vi "PUDELstat App.vi"() -> ()   [LabVIEW 2022 SP3]
doc: "PUDELstat App: a LabVIEW-based application to interface with and run electrochemistry experiments on the Potentiostat for Undergraduate-Designed Electrochemistry Laboratories. For more information, please visit www.eNanoLab.com/PUDELstat"
uses:
  Start.xctl
  Method Descriptions.xctl
  <vilib>/MakerHub/LINX/Public/Peripherals/PWM/PWM Set Duty Cycle 1 Chan.vi
  <vilib>/MakerHub/LINX/Public/Peripherals/Digital/Digital Read 1 Chan.vi
  <vilib>/MakerHub/LINX/Public/Peripherals/Digital/Digital Read N Chans.vi
  <vilib>/MakerHub/LINX/Private/Local IO/LinxDigitalRead.vi
  <vilib>/MakerHub/LINX/Public/Utilities/Check Channel.vi
  <vilib>/MakerHub/LINX/Public/Utilities/Open Serial.vi
  <vilib>/MakerHub/LINX/Public/Peripherals/PWM/PWM Set Duty Cycle N Chans.vi
  <vilib>/MakerHub/LINX/Private/Utilties/Generate Error.vi
  <vilib>/Utility/file.llb/Read Delimited Spreadsheet (DBL).vi
  <vilib>/Utility/file.llb/Write Delimited Spreadsheet (string).vi
  <vilib>/Utility/file.llb/Write Delimited Spreadsheet (DBL).vi
  <vilib>/MakerHub/LINX/LMH-LINX.lvlib
  <vilib>/Analysis/NI_AALPro.lvlib
panel:
  in  "Method Descriptions":bool(xcontrol)
  out "time (min)":dbl format="%#.1f"
  out "max time (min)":dbl format="%#.1f"
  out "Progress":dbl(slide) scale=0.0..30.1
  out "Current Limit":cluster{dbl, dbl}(slide)={0.001, 0.0} scale=-5.0..5.0 scale format="%_1f"
  in  "Save Path":path=path "C:/PUDELstat Data"
  in  "Method Selector":T1(tab)
  in  "Duration (s)\n[OCP]":dbl=30.0
  out "Open Circuit":cluster{dbl[], dbl[]}(graph)
  out "OCP (V)":dbl format="%#.2f"
  in  "Resolution (ms)\n[OCP]":dbl=100.0
  in  "Resolution (V)\n[CV]":dbl=0.02
  out "i (mA)\n[CV]":dbl format="%.2g"
  in  "Scan Rate (V/s)\n[CV]":dbl=0.1
  in  "Initial Potential (V)\n[CV]":dbl
  in  "First Vertex Potential (V)\n[CV]":dbl=1.0
  in  "Second Vertex Potential (V)\n[CV]":dbl=-1.0
  in  "Cycles\n[CV]":i32=1
  out "E (V)\n[CV]":dbl format="%.2g"
  out "Cyclic Voltammagram":cluster{dbl[], dbl[]}(graph)
  out "Applied and Response (CV)":T2(graph)
  in  "Final  Potential (V)\n[LSV]":dbl=1.0
  in  "Initial Potential (V)\n[LSV]":dbl
  in  "Scan Rate (V/s)\n[LSV]":dbl=0.1
  out "E (V)\n[lsv]":dbl format="%.2f"
  out "i (mA)\n[LSV]":dbl format="%.2f"
  out "Linear Sweep Voltammagram":cluster{dbl[], dbl[]}(graph)
  in  "Resolution (V)\n[LSV]":dbl=0.02
  out "Applied and Response (LSV)":T2(graph)
  in  "Scan Rate (V/s)\n[ASV]":dbl=0.1
  in  "Time (s)\n(standby)":dbl=30.0
  in  "Potential (V)\n(standby)":dbl
  in  "Final (V)\n[ASV]":dbl
  in  "Resolution (V)\n[ASV]":dbl=0.02
  in  "Time (s)\n(dep)":dbl=60.0
  in  "Potential (V)\n(dep)":dbl=-1.0
  in  "Time (s)\n(cleaning)":dbl=30.0
  in  "Potential (V)\n(cleaning)":dbl
  in  "Initial (V)\n[ASV)":dbl=-1.0
  out "Applied and Response (ASV)":T2(graph)
  out "E (V)\n[ASV]":dbl format="%.2f"
  out "i (mA)\n[ASV]":dbl format="%.2f"
  out "Anodic Stripping\n Voltammagram":cluster{dbl[], dbl[]}(graph)
  in  "Resolution (ms)\n[CA]":dbl=200.0
  out "i (mA)\n[CA]":dbl format="%.2f"
  out "q (C)":dbl format="%.2f"
  in  "Duration (s)\n[CA]":dbl=30.0
  in  "Set Potential (V)\n[CA]":dbl format="%#_13g"
  out "Chronoamperometry":cluster{dbl[], dbl[]}(graph)
  out "Energy Delivered (J)\n[CP]":dbl format="%.2f"
  out "P (mW)\n[CP]":dbl format="%.2f"
  in  "Potential (V)\n[CP]":dbl
  in  "Resolution (ms)\n[CP]":dbl=200.0
  out "E (V)\n[CP]":dbl format="%.2f"
  out "q (C)\n[CP]":dbl format="%.2f"
  in  "Duration (s)\n[CP]":dbl=10000.0
  in  "Set Current (mA)\n[CP]":dbl format="%#_13g"
  out "Chronopotentiometry":cluster{dbl[], dbl[]}(graph)
  out "E (V)\n[GC]":dbl format="%.2f"
  out "Galvanostatic Cycling":cluster{dbl[], dbl[]}(graph)
  in  "Set Current (mA)\n[GC]":dbl=5.0 format="%#_13g"
  in  "Duration (s)\n[GC]":dbl=30.0
  in  "Resolution (ms)\n[CP] 2":dbl=100.0
  in  "Measure Ru":bool=TRUE
  out "Ru (Ohm)":dbl format="%#.1f"
  in  "% Compensation":dbl=85.0
  out "Rc (Ohm)":dbl format="%#.1f"
  out "Eap (V)\n[iR]":dbl format="%.2f"
  out "i (mA)\n[iR]":dbl format="%.2f"
  in  "Cycles\n[iR]":i32=100
  in  "Pertubation Potential (V)":dbl=0.25
  in  "Resting Potential (V)":dbl format="%#_13g"
  in  "Frequency (mHz)\n[iR]":dbl=500.0 format="%#_13g"
  in  "Resolution (ms)\n[iR]":dbl=50.0
  out "Applied and Response (Ohmic)":T2(graph)
  in  "Potential Calibration":dbl[][](array[numeric])=[[0.954619, 0.02673]]
  in  "Current Calibration":dbl[][](array[numeric])=[[220.0, 4.99643, 0.11518, -10.0, 10.0], [510.0, 2.18568, 0.06108, -5.0, 5.0], [1000.0, 1.18065, 0.04067, -2.75, 2.75], [10000.0, 0.203334, 0.0077, -0.5, 0.5]]
  out "E Offset\n[Cal]":dbl format="%0.5f"
  out "R²\n[Calib] E":dbl format="%#_6f"
  out "E Conversion":dbl format="%#_6f"
  out "E Calibration":T3(graph)
  out "i Offset\n[Cal]":dbl format="%0.5f"
  out "R²\n[Calib] i":dbl format="%#_6f"
  out "i Conversion":dbl format="%#_6f"
  out "i Calibration":T3(graph)
  in  "Cycles \n[Cal]":i32=1
  in  "E2 (V)\n[Cal]":dbl=-1.0
  in  "E1 (V)\n[Cal]":dbl=1.0
  in  "Ei (V)\n[Cal]":dbl
  in  "Scan Rate (V/s)\n[Cal]":dbl=0.1
  in  "Sample Cell  Resistance (Ohm)":dbl=1000.0
  in  "Resolution (ms)\n[Cal]":dbl=100.0
  out "Applied and Response (Cal)":T2(graph)
  in  "Save Plot":u16(ring) items=["i vs E", "i vs t"]
  out "Preview (Single Cycle)":cluster{dbl[], "Preview":dbl[]}[](graph)
  in  "Element Selector":enum32{"A", "B", "C", "D", "E"}(tab) caption="Elements"
  in  "Input A":T4={"Element A"=0, "Scan Rate A"={"DE (V)\n[A]"=0.2, "Dt (s)\n[A]"=1.0}, "Input--Timing A"={"Duration (s)\n[MB-A]"=30.0, "Sample Rate (ms)\n[MB-A]"=100.0, "Frequency (mHz)\n[MB-A]"=1000.0, "Repeat n Times\n[MB-A]"=0}, "Input--Potential A"={"Ei (V)\n[A]"=0.0, "Ef (V)\n[A]"=1.0, "E1 (V)\n[A]"=1.0, "E2 (V)\n[A]"=-1.0, "Duty Cycle (%)\n[A]"=50.0}} {"Scan Rate A"."Dt (s)\n[A]" format="%0.2f"; "Scan Rate A"."DE (V)\n[A]" format="%0.2f"; "Element A" items=["Disabled", "Potentiostatic", "Linear Ramp", "Staircase Ramp", "Triangle Wave", "Square Wave", "Staircase Wave", "Sine Wave"]}
  in  "Input B":T5={"Element B"=0, "Input--Potential B"={"Ei (V)\n[B]"=0.0, "Ef (V)\n[B]"=1.0, "E1 (V)\n[B]"=1.0, "E2 (V)\n[B]"=-1.0, "Duty Cycle (%)\n[B]"=50.0}, "Input--Timing B"={"Duration (s)\n[MB-B]"=30.0, "Sample Rate (ms)\n[MB-B]"=100.0, "Frequency (mHz)\n[MB-B]"=1000.0, "Repeat n Times\n[MB-B]"=0}, "Scan Rate B"={"DE (V)\n[B]"=0.2, "Dt (s)\n[B]"=1.0}} {"Scan Rate B"."Dt (s)\n[B]" format="%0.2f"; "Scan Rate B"."DE (V)\n[B]" format="%0.2f"; "Element B" items=["Disabled", "Potentiostatic", "Linear Ramp", "Staircase Ramp", "Triangle Wave", "Square Wave", "Staircase Wave", "Sine Wave"]}
  in  "Input C":T6={"Scan Rate C"={"DE (V)\n[C]"=0.2, "Dt (s)\n[C]"=1.0}, "Input--Timing C"={"Duration (s)\n[MB-C]"=30.0, "Sample Rate (ms)\n[MB-C]"=100.0, "Frequency (mHz)\n[MB-C]"=1000.0, "Repeat n Times\n[MB-C]"=0}, "Input--Potential C"={"Ei (V)\n[C]"=0.0, "Ef (V)\n[C]"=1.0, "E1 (V)\n[C]"=1.0, "E2 (V)\n[C]"=-1.0, "Duty Cycle (%)\n[C]"=50.0}, "Element C"=0} {"Scan Rate C"."Dt (s)\n[C]" format="%0.2f"; "Scan Rate C"."DE (V)\n[C]" format="%0.2f"; "Element C" items=["Disabled", "Potentiostatic", "Linear Ramp", "Staircase Ramp", "Triangle Wave", "Square Wave", "Staircase Wave", "Sine Wave"]}
  in  "Input D":T7={"Scan Rate D"={"DE (V)\n[D]"=0.2, "Dt (s)\n[D]"=1.0}, "Input--Timing D"={"Duration (s)\n[MB-D]"=30.0, "Sample Rate (ms)\n[MB-D]"=100.0, "Frequency (mHz)\n[MB-D]"=1000.0, "Repeat n Times\n[MB-D]"=0}, "Input--Potential D"={"Ei (V)\n[D]"=0.0, "Ef (V)\n[D]"=1.0, "E1 (V)\n[D]"=1.0, "E2 (V)\n[D]"=-1.0, "Duty Cycle (%)\n[D]"=50.0}, "Element D"=0} {"Scan Rate D"."Dt (s)\n[D]" format="%0.2f"; "Scan Rate D"."DE (V)\n[D]" format="%0.2f"; "Element D" items=["Disabled", "Potentiostatic", "Linear Ramp", "Staircase Ramp", "Triangle Wave", "Square Wave", "Staircase Wave", "Sine Wave"]}
  in  "Input E":T8={"Scan Rate E"={"DE (V)\n[E]"=0.2, "Dt (s)\n[E]"=1.0}, "Input--Timing E"={"Duration (s)\n[MB-E]"=30.0, "Sample Rate (ms)\n[MB-E]"=100.0, "Frequency (mHz)\n[MB-E]"=1000.0, "Repeat n Times\n[MB-E]"=0}, "Input--Potential E"={"Ei (V)\n[E]"=0.0, "Ef (V)\n[E]"=1.0, "E1 (V)\n[E]"=1.0, "E2 (V)\n[E]"=-1.0, "Duty Cycle (%)\n[E]"=50.0}, "Element E"=0} {"Scan Rate E"."Dt (s)\n[E]" format="%0.2f"; "Scan Rate E"."DE (V)\n[E]" format="%0.2f"; "Element E" items=["Disabled", "Potentiostatic", "Linear Ramp", "Staircase Ramp", "Triangle Wave", "Square Wave", "Staircase Wave", "Sine Wave"]}
  in  "Mode":u16(ring) items=["Sequence: A->B->C->D->E", "Superimpose: A + B"]
  in  "Cycles\n[MB]":i32=1
  out "Signal Frequencies (mHz)":cluster{"A":dbl, "B":dbl}
  out "E (V)\nMB":dbl format="%.2f"
  out "i (mA)\n[MB]":dbl format="%.2f"
  out "Method i-t":cluster{dbl[], dbl[]}(graph)
  out "Method i-E":cluster{dbl[], dbl[]}(graph)
  out "R² \n[analysis]":dbl format="%#_6f"
  in  "Open Data":path
  in  "Plot Type":u16(ring) items=["Linear", "Tafel"]
  in  "E0 (V vs ref)":dbl
  out "Tafel Slope (mV/decade)":dbl
  out "i0 (mA)":dbl
  out "Analysis":cluster{"all rows":dbl[], "all rows":dbl[]}[](graph)
  in  "Cycle":dbl(ring)
  in  "Sensitivity (Jumper)":u16(ring)=1 items=["± 10 mA (220 Ohm)", "± 5 mA (510 Ohm)", "± 2.75 mA (1 kOhm)", "± 0.5 mA (10 kOhm)"]
  in  "Serial Port":refnum<visa-resource-name>="COM3"
  in  "Start":bool(xcontrol)
  in  "stop":bool
  # "/"
  # "(min)"
  # "Current Limits"
  # "Cleaning Step:"
  # "Deposition Step:"
  # "Stripping Step:"
  # "Standby:"
  # "Stop Condition:"
  # "or"
  # "E Conversion (measured/control)"
  # "E Offset (V)"
  # "Jumper (W)"
  # "i Conversion (mA/V)"
  # "i Offset (mA)"
  # "mHz"
  # "mHz"
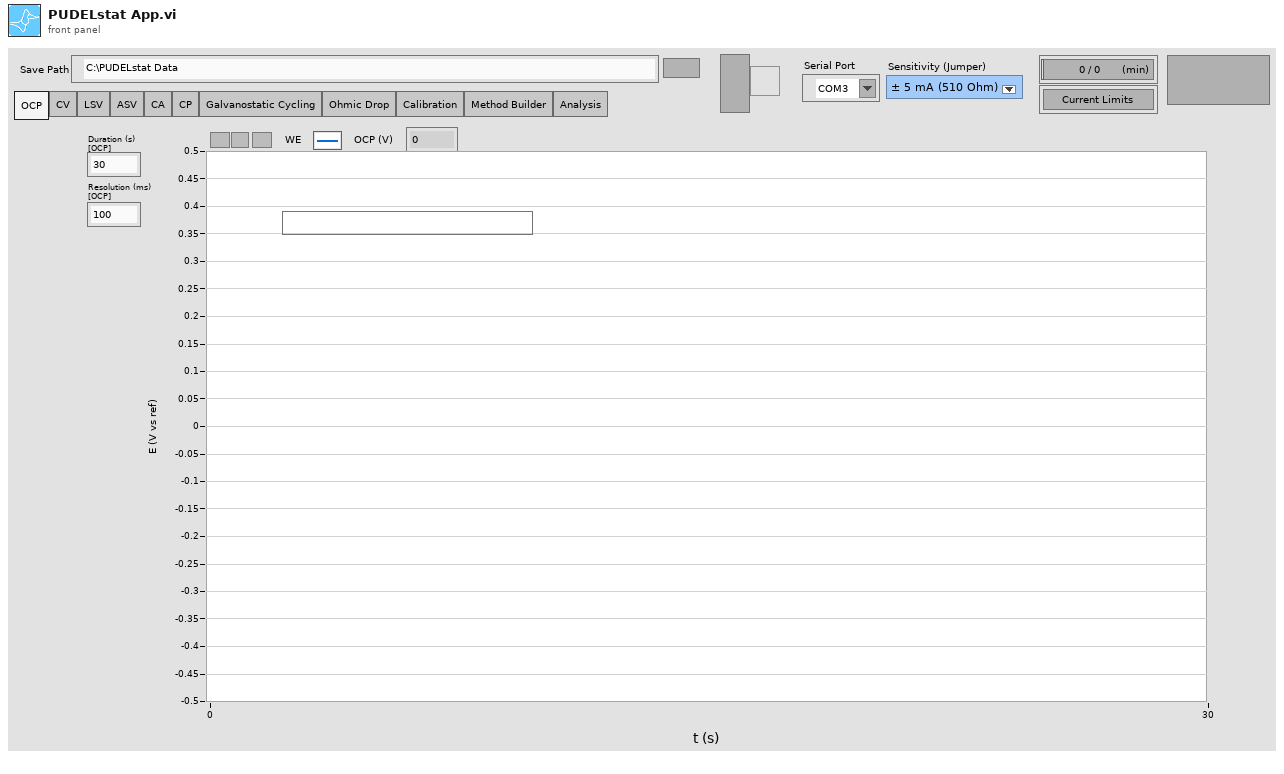
[diagram p1: front panel]
types:
  T1 = enum32{"OCP", "CV", "LSV", "ASV", "CA", "CP", "Galvanostatic Cycling", "Ohmic Drop", "Calibration", "Method Builder", "Analysis"}
  T2 = cluster{"Elapsed Time (s)":dbl[], "i (mA)":dbl[]}[]
  T3 = cluster{"Elapsed Time (s)":dbl[], "Best Linear Fit":dbl[]}[]
  T4 = cluster{"Element A":u16, "Scan Rate A":cluster{"DE (V)\n[A]":dbl, "Dt (s)\n[A]":dbl}, "Input--Timing A":cluster{"Duration (s)\n[MB-A]":dbl, "Sample Rate (ms)\n[MB-A]":dbl, "Frequency (mHz)\n[MB-A]":dbl, "Repeat n Times\n[MB-A]":i32}, "Input--Potential A":cluster{"Ei (V)\n[A]":dbl, "Ef (V)\n[A]":dbl, "E1 (V)\n[A]":dbl, "E2 (V)\n[A]":dbl, "Duty Cycle (%)\n[A]":dbl}}
  T5 = cluster{"Element B":u16, "Input--Potential B":cluster{"Ei (V)\n[B]":dbl, "Ef (V)\n[B]":dbl, "E1 (V)\n[B]":dbl, "E2 (V)\n[B]":dbl, "Duty Cycle (%)\n[B]":dbl}, "Input--Timing B":cluster{"Duration (s)\n[MB-B]":dbl, "Sample Rate (ms)\n[MB-B]":dbl, "Frequency (mHz)\n[MB-B]":dbl, "Repeat n Times\n[MB-B]":i32}, "Scan Rate B":cluster{"DE (V)\n[B]":dbl, "Dt (s)\n[B]":dbl}}
  T6 = cluster{"Scan Rate C":cluster{"DE (V)\n[C]":dbl, "Dt (s)\n[C]":dbl}, "Input--Timing C":cluster{"Duration (s)\n[MB-C]":dbl, "Sample Rate (ms)\n[MB-C]":dbl, "Frequency (mHz)\n[MB-C]":dbl, "Repeat n Times\n[MB-C]":i32}, "Input--Potential C":cluster{"Ei (V)\n[C]":dbl, "Ef (V)\n[C]":dbl, "E1 (V)\n[C]":dbl, "E2 (V)\n[C]":dbl, "Duty Cycle (%)\n[C]":dbl}, "Element C":u16}
  T7 = cluster{"Scan Rate D":cluster{"DE (V)\n[D]":dbl, "Dt (s)\n[D]":dbl}, "Input--Timing D":cluster{"Duration (s)\n[MB-D]":dbl, "Sample Rate (ms)\n[MB-D]":dbl, "Frequency (mHz)\n[MB-D]":dbl, "Repeat n Times\n[MB-D]":i32}, "Input--Potential D":cluster{"Ei (V)\n[D]":dbl, "Ef (V)\n[D]":dbl, "E1 (V)\n[D]":dbl, "E2 (V)\n[D]":dbl, "Duty Cycle (%)\n[D]":dbl}, "Element D":u16}
  T8 = cluster{"Scan Rate E":cluster{"DE (V)\n[E]":dbl, "Dt (s)\n[E]":dbl}, "Input--Timing E":cluster{"Duration (s)\n[MB-E]":dbl, "Sample Rate (ms)\n[MB-E]":dbl, "Frequency (mHz)\n[MB-E]":dbl, "Repeat n Times\n[MB-E]":i32}, "Input--Potential E":cluster{"Ei (V)\n[E]":dbl, "Ef (V)\n[E]":dbl, "E1 (V)\n[E]":dbl, "E2 (V)\n[E]":dbl, "Duty Cycle (%)\n[E]":dbl}, "Element E":u16}
  T9 = typedef "LMH-LINX.lvlib/LINX Ref.ctl" = cluster{"IO":T10, "Interface":T11, "LINX Device Config":T12}
  T10 = typedef "LMH-LINX.lvlib/Platform.ctl" = enum16{"Remote", "Local"}
  T11 = typedef "LMH-LINX.lvlib/Interface.ctl" = enum16{"Serial", "TCP"}
  T12 = typedef "LMH-LINX.lvlib/Device.lvlib/LINX Device Config.ctl" = cluster{"Interface":T11, "COM Port":refnum<visa-resource-name>, "TCP Configuration":T13, "Device Family":u8, "Device ID":u8, "Device Name":string, "TCP Ref":refnum<k5>, "Channels":T14}
  T13 = typedef "LMH-LINX.lvlib/Device.lvlib/TCP Config.ctl" = cluster{"IP Address":string, "Port":u16}
  T14 = typedef "LMH-LINX.lvlib/Channels.ctl" = cluster{"DI":u8[], "DO":u8[], "AI":u8[], "AO":u8[], "PWM":u8[], "QE":u8[], "UART":u8[], "I2C 2":u8[], "SPI":u8[], "CAN":u8[], "Servo":u8[], "AI Ref (V)":dbl, "AI Resolution (Bits)":u8, "AO Ref (V)":dbl, "AO Resolution (Bits)":u8}
  T15 = cluster{"Error Out":errorcluster, "LINX Resource":T9}
  T16 = cluster{"Signal Averaging?":bool, "CA?":bool, "Step Width":dbl}
  T17 = enum16{"Disabled", "Potentiostatic", "Linear Ramp", "Staircase Ramp", "Triangle Wave", "Square Wave", "Staircase Wave", "Sine Wave"}
  T18 = cluster{"Scan Rate D":cluster{"DE (V)":dbl, "Dt (s)":dbl}, "Input--Timing D":cluster{"Duration (s)":dbl, "Sample Rate (ms)":dbl, "Frequency (mHz)":dbl, "Repeat n Times":i32}, "Input--Potential D":cluster{"Ei (V)":dbl, "Ef (V)":dbl, "E1 (V)":dbl, "E2 (V)":dbl, "Duty Cycle (%)":dbl}, "Element D":u16}
  T19 = cluster{"Scan Rate C":cluster{"DE (V)":dbl, "Dt (s)":dbl}, "Input--Timing C":cluster{"Duration (s)":dbl, "Sample Rate (ms)":dbl, "Frequency (mHz)":dbl, "Repeat n Times":i32}, "Input--Potential C":cluster{"Ei (V)":dbl, "Ef (V)":dbl, "E1 (V)":dbl, "E2 (V)":dbl, "Duty Cycle (%)":dbl}, "Element C":u16}
  T20 = cluster{"Element B":u16, "Input--Potential B":cluster{"Ei (V)":dbl, "Ef (V)":dbl, "E1 (V)":dbl, "E2 (V)":dbl, "Duty Cycle (%)":dbl}, "Input--Timing B":cluster{"Duration (s)":dbl, "Sample Rate (ms)":dbl, "Frequency (mHz)":dbl, "Repeat n Times":i32}, "Scan Rate B":cluster{"DE (V)":dbl, "Dt (s)":dbl}}
  T21 = cluster{"Element A":u16, "Scan Rate A":cluster{"DE (V)":dbl, "Dt (s)":dbl}, "Input--Timing A":cluster{"Duration (s)":dbl, "Sample Rate (ms)":dbl, "Frequency (mHz)":dbl, "Repeat n Times":i32}, "Input--Potential A":cluster{"Ei (V)":dbl, "Ef (V)":dbl, "E1 (V)":dbl, "E2 (V)":dbl, "Duty Cycle (%)":dbl}}
  T22 = cluster{"Duty Cycle Array":dbl[], "Wait Time (ms)":dbl, "Array Size":i32, "Frequency (mHz)":dbl, "Corrected Duty Cycle Array":dbl[], "Potential Array":dbl[]}
  T23 = cluster{dbl[], "Resolution (ms)\n[OCP]":dbl, i32, dbl, dbl[], dbl[]}
  T24 = cluster{"Initial Potential (V)\n[CV]":dbl, dbl, "First Vertex Potential (V)\n[CV]":dbl, "Second Vertex Potential (V)\n[CV]":dbl, dbl}
  T25 = cluster{"Initial Potential (V)\n[LSV]":dbl, "Final  Potential (V)\n[LSV]":dbl, dbl, dbl, dbl}
  T26 = cluster{"Duration (s)\n[CA]":dbl, "Resolution (ms)\n[CA]":dbl, dbl, i32}
  T27 = cluster{"Set Potential (V)\n[CA]":dbl, dbl, dbl, dbl, dbl}
  T28 = cluster{"Duration (s)\n[CP]":dbl, "Resolution (ms)\n[CP]":dbl, dbl, i32}
  T29 = cluster{"Resting Potential (V)":dbl, "Pertubation Potential (V)":dbl, dbl, dbl, dbl}
  T30 = cluster{dbl, "Resolution (ms)\n[iR]":dbl, "Frequency (mHz)\n[iR]":dbl, i32}
  T31 = cluster{"Ei (V)\n[Cal]":dbl, dbl, "E1 (V)\n[Cal]":dbl, "E2 (V)\n[Cal]":dbl, dbl}
  T32 = cluster{dbl, "Resolution (ms)\n[Cal]":dbl, dbl, i32}
  T33 = cluster{"Elapsed Time (s)":dbl[], "E (V)":dbl[], "i (mA)":dbl[], "Vr (V)":dbl[], "Eraw (V)":dbl[]}
  T34 = cluster{"Wait Time (ms)":dbl, i32, "Array Size":i32, u32}
  T35 = cluster{"Elapsed Time (s)":dbl[], "i (mA)":dbl[]}
  T36 = cluster{"Elapsed Time (s)":dbl[], "Eraw (V)":dbl[]}
  T37 = cluster{"error out":errorcluster, "LINX Resource out":T9}
  T38 = cluster{"E (V)":dbl[], "Best Linear Fit":dbl[]}[]
  T39 = cluster{"Eraw (V)":dbl[], "Best Linear Fit":dbl[]}
  T40 = cluster{"Eraw (V)":dbl[], "Best Linear Fit":dbl[]}[]
  T41 = cluster{"error out":errorcluster, "LINX Resource":T9}
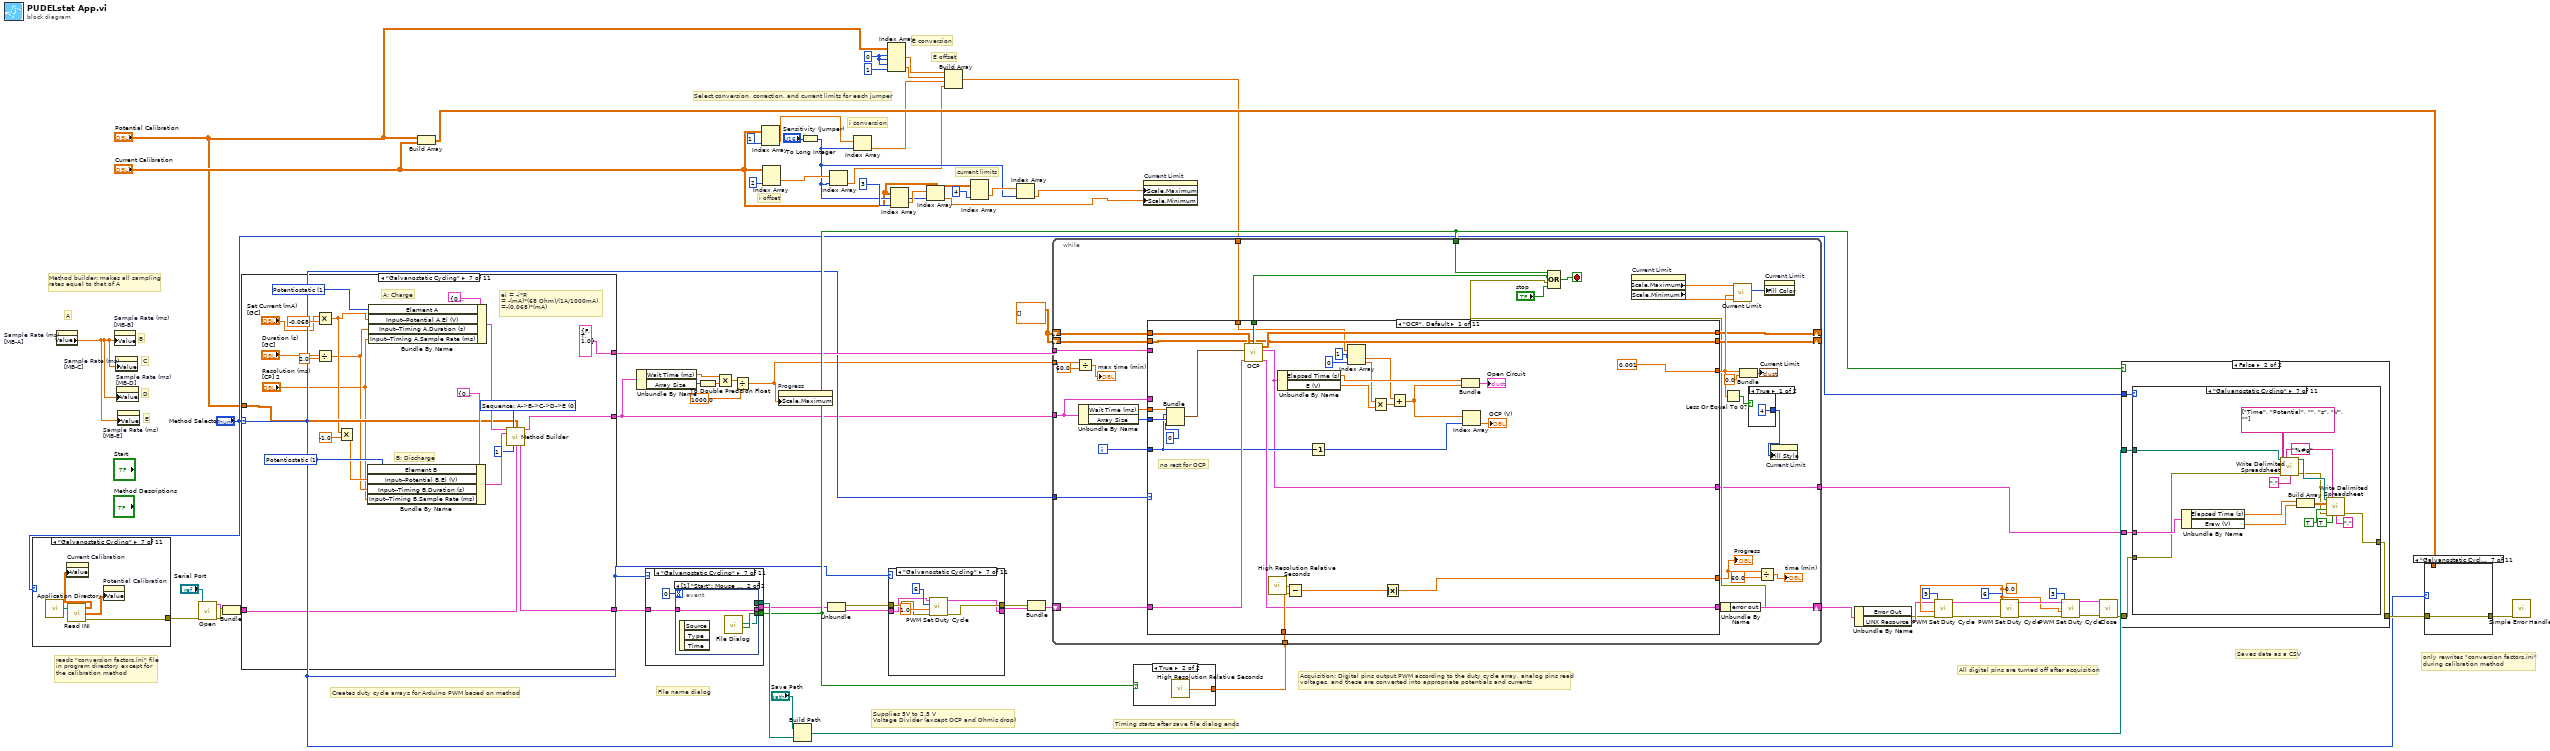
[diagram p0: block diagram]
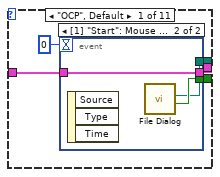
[diagram p2: hidden frame]
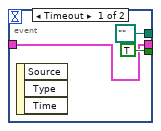
[diagram p3: hidden frame]
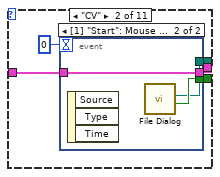
[diagram p4: hidden frame]
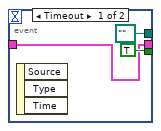
[diagram p5: hidden frame]
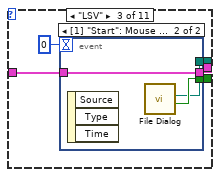
[diagram p6: hidden frame]
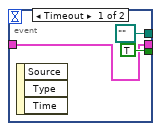
[diagram p7: hidden frame]
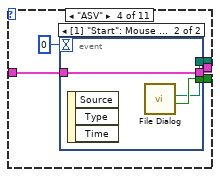
[diagram p8: hidden frame]
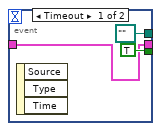
[diagram p9: hidden frame]
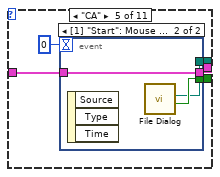
[diagram p10: hidden frame]
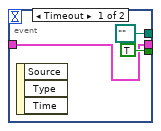
[diagram p11: hidden frame]
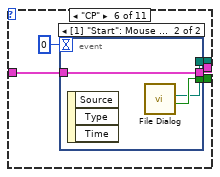
[diagram p12: hidden frame]
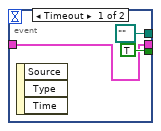
[diagram p13: hidden frame]
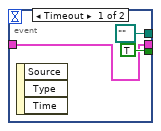
[diagram p14: hidden frame]
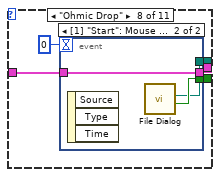
[diagram p15: hidden frame]
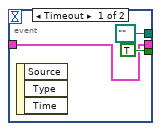
[diagram p16: hidden frame]
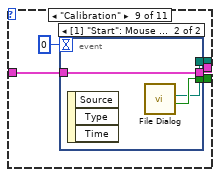
[diagram p17: hidden frame]
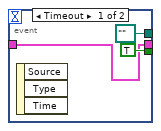
[diagram p18: hidden frame]
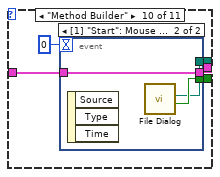
[diagram p19: hidden frame]
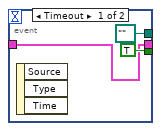
[diagram p20: hidden frame]
diagram:
  w7 = 0 ("index (row)")
  w29 = dbl[][] [] ("Data Out")
  w46 = 0.0 ("Duty Cycle (0-1)")
  # "E offset"
  # "E conversion"
  # "current limits"
  # "i offset"
  # "i conversion"
  # "Select conversion, correction, and current limits for each jumper"
  # "Saves data as a CSV"
  # "All digital pins are turned off after acquisition"
  # "Acquisition: Digital pins output PWM according to the duty cycle array, analog pins read\nvoltages, and these are converted into appropriate potentials and currents"
  # "File name dialog"
  # "Creates duty cycle arrays for Arduino PWM based on method"
  # "Supplies 5V to 2.5 V\nVoltage Divider (except OCP and Ohmic drop)"
  # "only rewrites \"conversion factors.ini\"\nduring calibration method"
  # "reads \"conversion factors.ini\" file\nin program directory except for\nthe calibration method"
  # "Timing starts after save file dialog ends"
  # "Method builder: makes all sampling\nrates equal to that of A"
  # "E"
  # "D"
  # "C"
  # "B"
  # "A"
  n1 = case shown="\"Galvanostatic Cycling\"" "Method Selector" {
    tunnel: [w69 w73 w77 w81 w85 w89 w93 w97 errorcluster {"status"=FALSE, "code"=0, "source"=""} ("error out") w102 w106] -> w32
    frame "OCP", Default {
      n2 = call <vilib>:"Application Directory.vi"() -> ("Application Directory"=w70:path)
      n3 = call "Read INI.vi"("Path"=w70) -> ("Current Calibration"=w71:dbl[][], "Voltage Calibration"=w68:dbl[][], "error out"=w69:errorcluster)  [unwired: 1 in]
      n4 = property on="Current Calibration" class="Arr (strict)"("Value"=w71) -> ()  [unwired: 2 in, 2 out]
      n5 = property on="Potential Calibration" class="Arr (strict)"("Value"=w68) -> ()  [unwired: 2 in, 2 out]
    }
    frame "CV" {
      n6 = call <vilib>:"Application Directory.vi"() -> ("Application Directory"=w74:path)
      n7 = call "Read INI.vi"("Path"=w74) -> ("Current Calibration"=w75:dbl[][], "Voltage Calibration"=w72:dbl[][], "error out"=w73:errorcluster)  [unwired: 1 in]
      n8 = property on="Current Calibration" class="Arr (strict)"("Value"=w75) -> ()  [unwired: 2 in, 2 out]
      n9 = property on="Potential Calibration" class="Arr (strict)"("Value"=w72) -> ()  [unwired: 2 in, 2 out]
    }
    frame "LSV" {
      n10 = call <vilib>:"Application Directory.vi"() -> ("Application Directory"=w78:path)
      n11 = call "Read INI.vi"("Path"=w78) -> ("Current Calibration"=w79:dbl[][], "Voltage Calibration"=w76:dbl[][], "error out"=w77:errorcluster)  [unwired: 1 in]
      n12 = property on="Current Calibration" class="Arr (strict)"("Value"=w79) -> ()  [unwired: 2 in, 2 out]
      n13 = property on="Potential Calibration" class="Arr (strict)"("Value"=w76) -> ()  [unwired: 2 in, 2 out]
    }
    frame "ASV" {
      n14 = call <vilib>:"Application Directory.vi"() -> ("Application Directory"=w82:path)
      n15 = call "Read INI.vi"("Path"=w82) -> ("Current Calibration"=w83:dbl[][], "Voltage Calibration"=w80:dbl[][], "error out"=w81:errorcluster)  [unwired: 1 in]
      n16 = property on="Current Calibration" class="Arr (strict)"("Value"=w83) -> ()  [unwired: 2 in, 2 out]
      n17 = property on="Potential Calibration" class="Arr (strict)"("Value"=w80) -> ()  [unwired: 2 in, 2 out]
    }
    frame "CA" {
      n18 = call <vilib>:"Application Directory.vi"() -> ("Application Directory"=w86:path)
      n19 = call "Read INI.vi"("Path"=w86) -> ("Current Calibration"=w87:dbl[][], "Voltage Calibration"=w84:dbl[][], "error out"=w85:errorcluster)  [unwired: 1 in]
      n20 = property on="Current Calibration" class="Arr (strict)"("Value"=w87) -> ()  [unwired: 2 in, 2 out]
      n21 = property on="Potential Calibration" class="Arr (strict)"("Value"=w84) -> ()  [unwired: 2 in, 2 out]
    }
    frame "CP" {
      n22 = call <vilib>:"Application Directory.vi"() -> ("Application Directory"=w90:path)
      n23 = call "Read INI.vi"("Path"=w90) -> ("Current Calibration"=w91:dbl[][], "Voltage Calibration"=w88:dbl[][], "error out"=w89:errorcluster)  [unwired: 1 in]
      n24 = property on="Current Calibration" class="Arr (strict)"("Value"=w91) -> ()  [unwired: 2 in, 2 out]
      n25 = property on="Potential Calibration" class="Arr (strict)"("Value"=w88) -> ()  [unwired: 2 in, 2 out]
    }
    frame "Galvanostatic Cycling" {
      n26 = call <vilib>:"Application Directory.vi"() -> ("Application Directory"=w94:path)
      n27 = call "Read INI.vi"("Path"=w94) -> ("Current Calibration"=w95:dbl[][], "Voltage Calibration"=w92:dbl[][], "error out"=w93:errorcluster)  [unwired: 1 in]
      n28 = property on="Current Calibration" class="Arr (strict)"("Value"=w95) -> ()  [unwired: 2 in, 2 out]
      n29 = property on="Potential Calibration" class="Arr (strict)"("Value"=w92) -> ()  [unwired: 2 in, 2 out]
    }
    frame "Ohmic Drop" {
      n30 = call <vilib>:"Application Directory.vi"() -> ("Application Directory"=w98:path)
      n31 = call "Read INI.vi"("Path"=w98) -> ("Current Calibration"=w99:dbl[][], "Voltage Calibration"=w96:dbl[][], "error out"=w97:errorcluster)  [unwired: 1 in]
      n32 = property on="Current Calibration" class="Arr (strict)"("Value"=w99) -> ()  [unwired: 2 in, 2 out]
      n33 = property on="Potential Calibration" class="Arr (strict)"("Value"=w96) -> ()  [unwired: 2 in, 2 out]
    }
    frame "Calibration" {
    }
    frame "Method Builder" {
      n34 = call <vilib>:"Application Directory.vi"() -> ("Application Directory"=w103:path)
      n35 = call "Read INI.vi"("Path"=w103) -> ("Current Calibration"=w104:dbl[][], "Voltage Calibration"=w101:dbl[][], "error out"=w102:errorcluster)  [unwired: 1 in]
      n36 = property on="Current Calibration" class="Arr (strict)"("Value"=w104) -> ()  [unwired: 2 in, 2 out]
      n37 = property on="Potential Calibration" class="Arr (strict)"("Value"=w101) -> ()  [unwired: 2 in, 2 out]
    }
    frame "Analysis" {
      n38 = call <vilib>:"Application Directory.vi"() -> ("Application Directory"=w107:path)
      n39 = call "Read INI.vi"("Path"=w107) -> ("Current Calibration"=w108:dbl[][], "Voltage Calibration"=w105:dbl[][], "error out"=w106:errorcluster)  [unwired: 1 in]
      n40 = property on="Current Calibration" class="Arr (strict)"("Value"=w108) -> ()  [unwired: 2 in, 2 out]
      n41 = property on="Potential Calibration" class="Arr (strict)"("Value"=w105) -> ()  [unwired: 2 in, 2 out]
    }
  }
  n42 = property on="Sample Rate (ms)\n[MB-A]" class="DigNum (strict)"() -> ("Value"=w35:dbl)  [unwired: 2 in, 2 out]
  n43 = property on="Sample Rate (ms)\n[MB-B]" class="DigNum (strict)"("Value"=w35) -> ()  [unwired: 2 in, 2 out]
  n44 = property on="Sample Rate (ms)\n[MB-C]" class="DigNum (strict)"("Value"=w35) -> ()  [unwired: 2 in, 2 out]
  n45 = property on="Sample Rate (ms)\n[MB-D]" class="DigNum (strict)"("Value"=w35) -> ()  [unwired: 2 in, 2 out]
  n46 = property on="Sample Rate (ms)\n[MB-E]" class="DigNum (strict)"("Value"=w35) -> ()  [unwired: 2 in, 2 out]
  n47 = call-poly <vilib>:"Open.vi"("Error In"=w32, "Serial Port"="Serial Port") -> ("Error Out"=w44:errorcluster, "LINX Resource"=w43:T9)  [unwired: 7 in, 1 out]
  n48 = Bundle("Error Out"=w44, "LINX Resource"=w43) -> (w42:T15)  [unwired: 1 in]
  n49 = case shown="\"Galvanostatic Cycling\"" "Method Selector" {
    tunnel: w42 -> [w120 w140 w166 w184 w218 w232 w246 w263 w280 w296 w308]
    tunnel: [w120 w139 w165 w183 w217 w231 w247 w262 w279 w295 w308] -> w22
    tunnel: [w111 w123 w164 w173 w212 w233 w249 w264 w278 w294 T22 {"Duty Cycle Array"=[], "Wait Time (ms)"=0.0, "Array Size"=0, "Frequency (mHz)"=0.0, "Corrected Duty Cycle Array"=[], "Potential Array"=[]} ("Output")] -> w11
    tunnel: [T16 {"Signal Averaging?"=FALSE, "CA?"=FALSE, "Step Width"=1.0} ("Averaging and Conversion") w137 w162 w206 T16 {"Signal Averaging?"=FALSE, "CA?"=TRUE, "Step Width"=1.0} ("Averaging and Conversion") T16 {"Signal Averaging?"=FALSE, "CA?"=TRUE, "Step Width"=1.0} ("Averaging and Conversion") T16 {"Signal Averaging?"=FALSE, "CA?"=TRUE, "Step Width"=1.0} ("Averaging and Conversion") T16 {"Signal Averaging?"=FALSE, "CA?"=FALSE, "Step Width"=1.0} ("Averaging and Conversion") T16 {"Signal Averaging?"=FALSE, "CA?"=FALSE, "Step Width"=1.0} ("Averaging and Conversion") T16 {"Signal Averaging?"=FALSE, "CA?"=FALSE, "Step Width"=1.0} ("Averaging and Conversion") T16 {"Signal Averaging?"=FALSE, "CA?"=FALSE, "Step Width"=0.0} ("Averaging and Conversion")] -> w28
    tunnel: "Potential Calibration" -> [_ w121 w147 w174 w208 w221 w248 w258 w274 w292 _]
    frame "OCP", Default {
      w109 = dbl[] []
      # "Samples = Duration/resolution\n+1 (for spurious first pt)"
      n50 = Multiply(x=1000.0, y="Duration (s)\n[OCP]") -> (x*y=w118:dbl)
      n51 = Divide(x=w118, y="Resolution (ms)\n[OCP]") -> (x/y=w117:dbl)
      n52 = Increment(x=w117) -> (x+1=w116:dbl)
      n53 = To Long Integer(number=w116) -> (32bit integer=w113:i32)
      n54 = Bundle(w109, "Resolution (ms)\n[OCP]"="Resolution (ms)\n[OCP]", w113, 0.0, w109, w109) -> (w111:T23)  [unwired: 1 in]
    }
    frame "CV" {
      w132 = 20.0 ("Resolution (ms)")
      w124 = 0.0
      # "20 ms sampling (50 Hz)"
      n55 = Decrement(x="Cycles\n[CV]") -> (x-1=w142:i32)
      n56 = Divide(x="Resolution (V)\n[CV]", y="Scan Rate (V/s)\n[CV]") -> (x/y=w128:dbl)
      n57 = Bundle By Name(cluster=cluster{"DE (V)":dbl, "Dt (s)":dbl} {"DE (V)"=1.0, "Dt (s)"=1.0} ("Input--Scan Rate"), "DE (V)"="Resolution (V)\n[CV]", "Dt (s)"=w128) -> (w126:cluster{"DE (V)":dbl, "Dt (s)":dbl})
      n58 = Bundle("Initial Potential (V)\n[CV]"="Initial Potential (V)\n[CV]", w124, "First Vertex Potential (V)\n[CV]"="First Vertex Potential (V)\n[CV]", "Second Vertex Potential (V)\n[CV]"="Second Vertex Potential (V)\n[CV]", w124) -> (w144:T24)  [unwired: 1 in]
      n59 = Bundle(w124, "Resolution (ms)"=w132, w124, w142) -> (w141:cluster{dbl, "Resolution (ms)":dbl, dbl, i32})  [unwired: 1 in]
      n60 = Divide(x=w132, y=1000.0) -> (x/y=w133:dbl)
      n61 = Divide(x=w128, y=w133) -> (x/y=w127:dbl)
      n62 = call "Method Elements.vi"("Arduino In"=w140, "Potential Calibration"=w121, "Input--Scan Rate"=w126, "Input--Timing"=w141, "Input--Potential"=w144, "Element"=T17."Staircase Wave") -> ("Output"=w123:T22, "Arduino Out"=w139:cluster{"Error Out":errorcluster, "LINX Out":T9})  [unwired: 4 in]
      n63 = Bundle By Name(cluster=T16 {"Signal Averaging?"=TRUE, "CA?"=FALSE, "Step Width"=0.0} ("Averaging and Conversion"), "Signal Averaging?"=TRUE ("Signal Averaging? 2"), "CA?"=FALSE ("Signal Averaging? 2"), "Step Width"=w127) -> (w137:T16)
    }
    frame "LSV" {
      w151 = 20.0
      w167 = 0.0
      # "20 ms sampling (50 Hz)"
      n64 = Divide(x="Resolution (V)\n[LSV]", y="Scan Rate (V/s)\n[LSV]") -> (x/y=w152:dbl)
      n65 = Bundle(w167, w151, w167, 0) -> (w159:cluster{dbl, dbl, dbl, i32})  [unwired: 1 in]
      n66 = Bundle("Initial Potential (V)\n[LSV]"="Initial Potential (V)\n[LSV]", "Final  Potential (V)\n[LSV]"="Final  Potential (V)\n[LSV]", w167, w167, w167) -> (w169:T25)  [unwired: 1 in]
      n67 = Bundle By Name(cluster=cluster{"DE (V)":dbl, "Dt (s)":dbl} {"DE (V)"=1.0, "Dt (s)"=1.0} ("Input--Scan Rate"), "DE (V)"="Resolution (V)\n[LSV]", "Dt (s)"=w152) -> (w155:cluster{"DE (V)":dbl, "Dt (s)":dbl})
      n68 = Divide(x=w151, y=1000.0) -> (x/y=w153:dbl)
      n69 = Divide(x=w152, y=w153) -> (x/y=w150:dbl)
      n70 = call "Method Elements.vi"("Arduino In"=w166, "Potential Calibration"=w147, "Input--Scan Rate"=w155, "Input--Timing"=w159, "Input--Potential"=w169, "Element"=T17."Staircase Ramp") -> ("Output"=w164:T22, "Arduino Out"=w165:cluster{"Error Out":errorcluster, "LINX Out":T9})  [unwired: 4 in]
      n71 = Bundle By Name(cluster=T16 {"Signal Averaging?"=TRUE, "CA?"=FALSE, "Step Width"=0.0} ("Averaging and Conversion"), "Signal Averaging?"=TRUE, "CA?"=FALSE, "Step Width"=w150) -> (w162:T16)
    }
    frame "ASV" {
      w182 = u16 1 items=["Disabled", "Potentiostatic", "Linear Ramp", "Staircase Ramp", "Triangle Wave", "Square Wave", "Staircase Wave", "Sine Wave"] ("Element A")
      w191 = u16 3 items=["Disabled", "Potentiostatic", "Linear Ramp", "Staircase Ramp", "Triangle Wave", "Square Wave", "Staircase Wave", "Sine Wave"] ("Element A")
      w197 = u16 1 items=["Disabled", "Potentiostatic", "Linear Ramp", "Staircase Ramp", "Triangle Wave", "Square Wave", "Staircase Wave", "Sine Wave"] ("Element A")
      w171 = 20.0 ("Input--Timing A.Sample Rate (ms)")
      w201 = u16 1 items=["Disabled", "Potentiostatic", "Linear Ramp", "Staircase Ramp", "Triangle Wave", "Square Wave", "Staircase Wave", "Sine Wave"] ("Element A")
      w203 = u16 0 items=["Sequence: A->B->C->D->E", "Superimpose: A + B"] ("Mode")
      # "D: Standby"
      # "C: Stripping"
      # "B: Deposition"
      # "A: Cleaning"
      # "20 ms sampling (50 Hz)"
      n72 = Divide(x="Resolution (V)\n[ASV]", y="Scan Rate (V/s)\n[ASV]") -> (x/y=w178:dbl)
      n73 = Bundle By Name(cluster=T21 {"Element A"=0, "Scan Rate A"={"DE (V)"=0.2, "Dt (s)"=1.0}, "Input--Timing A"={"Duration (s)"=30.0, "Sample Rate (ms)"=100.0, "Frequency (mHz)"=1000.0, "Repeat n Times"=0}, "Input--Potential A"={"Ei (V)"=0.0, "Ef (V)"=1.0, "E1 (V)"=1.0, "E2 (V)"=-1.0, "Duty Cycle (%)"=50.0}} ("Input A"), "Element A"=w201, "Input--Potential A.Ei (V)"="Potential (V)\n(cleaning)", "Input--Timing A.Duration (s)"="Time (s)\n(cleaning)", "Input--Timing A.Sample Rate (ms)"=w171) -> (w194:T21)
      n74 = Bundle By Name(cluster=T20 {"Element B"=0, "Input--Potential B"={"Ei (V)"=0.0, "Ef (V)"=1.0, "E1 (V)"=1.0, "E2 (V)"=-1.0, "Duty Cycle (%)"=50.0}, "Input--Timing B"={"Duration (s)"=30.0, "Sample Rate (ms)"=100.0, "Frequency (mHz)"=1000.0, "Repeat n Times"=0}, "Scan Rate B"={"DE (V)"=0.2, "Dt (s)"=1.0}} ("Input B"), "Element B"=w197, "Input--Potential B.Ei (V)"="Potential (V)\n(dep)", "Input--Timing B.Duration (s)"="Time (s)\n(dep)", "Input--Timing B.Sample Rate (ms)"=w171) -> (w193:T20)
      n75 = Bundle By Name(cluster=T18 {"Scan Rate D"={"DE (V)"=0.2, "Dt (s)"=1.0}, "Input--Timing D"={"Duration (s)"=30.0, "Sample Rate (ms)"=100.0, "Frequency (mHz)"=1000.0, "Repeat n Times"=0}, "Input--Potential D"={"Ei (V)"=0.0, "Ef (V)"=1.0, "E1 (V)"=1.0, "E2 (V)"=-1.0, "Duty Cycle (%)"=50.0}, "Element D"=0} ("Input D"), "Element D"=w182, "Input--Potential D.Ei (V)"="Potential (V)\n(standby)", "Input--Timing D.Duration (s)"="Time (s)\n(standby)", "Input--Timing D.Sample Rate (ms)"=w171) -> (w176:T18)
      n76 = Bundle By Name(cluster=T19 {"Scan Rate C"={"DE (V)"=0.2, "Dt (s)"=1.0}, "Input--Timing C"={"Duration (s)"=30.0, "Sample Rate (ms)"=100.0, "Frequency (mHz)"=1000.0, "Repeat n Times"=0}, "Input--Potential C"={"Ei (V)"=0.0, "Ef (V)"=1.0, "E1 (V)"=1.0, "E2 (V)"=-1.0, "Duty Cycle (%)"=50.0}, "Element C"=0} ("Input C"), "Element C"=w191, "Input--Potential C.Ei (V)"="Initial (V)\n[ASV)", "Input--Potential C.Ef (V)"="Final (V)\n[ASV]", "Scan Rate C.DE (V)"="Resolution (V)\n[ASV]", "Scan Rate C.Dt (s)"=w178, "Input--Timing C.Sample Rate (ms)"=w171) -> (w186:T19)
      n77 = call "Method Builder.vi"("Input A"=w194, "Mode"=w203, "Potential Calibration"=w174, "Input B"=w193, "Input C"=w186, "Input D"=w176, "Cycles"=1, "Arduino In"=w184) -> ("Output"=w173:T22, "Arduino Out"=w183:cluster{"Error Out":errorcluster, "LINX Out":T9})  [unwired: 4 in, 2 out]
      n78 = Divide(x=w171, y=1000.0) -> (x/y=w179:dbl)
      n79 = Divide(x=w178, y=w179) -> (x/y=w177:dbl)
      n80 = Bundle By Name(cluster=T16 {"Signal Averaging?"=TRUE, "CA?"=FALSE, "Step Width"=0.0} ("Averaging and Conversion"), "Signal Averaging?"=TRUE ("Signal Averaging? 2"), "CA?"=FALSE ("Signal Averaging? 2"), "Step Width"=w177) -> (w206:T16)
    }
    frame "CA" {
      w210 = 0.0
      n81 = Bundle("Duration (s)\n[CA]"="Duration (s)\n[CA]", "Resolution (ms)\n[CA]"="Resolution (ms)\n[CA]", w210, 0) -> (w213:T26)  [unwired: 1 in]
      n82 = Bundle("Set Potential (V)\n[CA]"="Set Potential (V)\n[CA]", w210, w210, w210, w210) -> (w219:T27)  [unwired: 1 in]
      n83 = call "Method Elements.vi"("Arduino In"=w218, "Potential Calibration"=w208, "Input--Timing"=w213, "Input--Potential"=w219, "Element"=T17."Potentiostatic") -> ("Output"=w212:T22, "Arduino Out"=w217:cluster{"Error Out":errorcluster, "LINX Out":T9})  [unwired: 5 in]
    }
    frame "CP" {
      w229 = 0.0
      # "ei = -i*R\n= -(mA)*(68 Ohm)/(1A/1000mA)\n=-(0.068)*(mA)"
      n84 = Multiply(x="Set Current (mA)\n[CP]", y=-0.068) -> (x*y=w227:dbl)
      n85 = Bundle("Duration (s)\n[CP]"="Duration (s)\n[CP]", "Resolution (ms)\n[CP]"="Resolution (ms)\n[CP]", w229, 0) -> (w222:T28)  [unwired: 1 in]
      n86 = Bundle(w227, w229, w229, w229, w229) -> (w225:cluster{dbl, dbl, dbl, dbl, dbl})  [unwired: 1 in]
      n87 = call "Method Elements.vi"("Arduino In"=w232, "Potential Calibration"=w221, "Input--Timing"=w222, "Input--Potential"=w225, "Element"=T17."Potentiostatic") -> ("Output"=w233:T22, "Arduino Out"=w231:cluster{"Error Out":errorcluster, "LINX Out":T9})  [unwired: 5 in]
    }
    frame "Galvanostatic Cycling" {
      w253 = u16 1 items=["Disabled", "Potentiostatic", "Linear Ramp", "Staircase Ramp", "Triangle Wave", "Square Wave", "Staircase Wave", "Sine Wave"] ("Element A")
      w255 = u16 1 items=["Disabled", "Potentiostatic", "Linear Ramp", "Staircase Ramp", "Triangle Wave", "Square Wave", "Staircase Wave", "Sine Wave"] ("Element A")
      w257 = u16 0 items=["Sequence: A->B->C->D->E", "Superimpose: A + B"] ("Mode")
      # "ei = -i*R\n= -(mA)*(68 Ohm)/(1A/1000mA)\n=-(0.068)*(mA)"
      # "B: Discharge"
      # "A: Charge"
      n88 = Multiply(x="Set Current (mA)\n[GC]", y=-0.068) -> (x*y=w240:dbl)
      n89 = Divide(x="Duration (s)\n[GC]", y=2.0) -> (x/y=w237:dbl)
      n90 = Multiply(x=w240, y=-1.0) -> (x*y=w239:dbl)
      n91 = Bundle By Name(cluster=T20 {"Element B"=0, "Input--Potential B"={"Ei (V)"=0.0, "Ef (V)"=1.0, "E1 (V)"=1.0, "E2 (V)"=-1.0, "Duty Cycle (%)"=50.0}, "Input--Timing B"={"Duration (s)"=30.0, "Sample Rate (ms)"=100.0, "Frequency (mHz)"=1000.0, "Repeat n Times"=0}, "Scan Rate B"={"DE (V)"=0.2, "Dt (s)"=1.0}} ("Input B"), "Element B"=w253, "Input--Potential B.Ei (V)"=w239, "Input--Timing B.Duration (s)"=w237, "Input--Timing B.Sample Rate (ms)"="Resolution (ms)\n[CP] 2") -> (w251:T20)
      n92 = Bundle By Name(cluster=T21 {"Element A"=0, "Scan Rate A"={"DE (V)"=0.2, "Dt (s)"=1.0}, "Input--Timing A"={"Duration (s)"=30.0, "Sample Rate (ms)"=100.0, "Frequency (mHz)"=1000.0, "Repeat n Times"=0}, "Input--Potential A"={"Ei (V)"=0.0, "Ef (V)"=1.0, "E1 (V)"=1.0, "E2 (V)"=-1.0, "Duty Cycle (%)"=50.0}} ("Input A"), "Element A"=w255, "Input--Potential A.Ei (V)"=w240, "Input--Timing A.Duration (s)"=w237, "Input--Timing A.Sample Rate (ms)"="Resolution (ms)\n[CP] 2") -> (w252:T21)
      n93 = call "Method Builder.vi"("Input A"=w252, "Mode"=w257, "Potential Calibration"=w248, "Input B"=w251, "Cycles"=1, "Arduino In"=w246) -> ("Output"=w249:T22, "Arduino Out"=w247:cluster{"Error Out":errorcluster, "LINX Out":T9})  [unwired: 6 in, 2 out]
    }
    frame "Ohmic Drop" {
      w267 = 0.0
      n94 = Decrement(x="Cycles\n[iR]") -> (x-1=w272:i32)
      n95 = Bundle("Resting Potential (V)"="Resting Potential (V)", "Pertubation Potential (V)"="Pertubation Potential (V)", w267, w267, 50.0) -> (w265:T29)  [unwired: 1 in]
      n96 = Bundle(w267, "Resolution (ms)\n[iR]"="Resolution (ms)\n[iR]", "Frequency (mHz)\n[iR]"="Frequency (mHz)\n[iR]", w272) -> (w271:T30)  [unwired: 1 in]
      n97 = call "Method Elements.vi"("Arduino In"=w263, "Potential Calibration"=w258, "Input--Timing"=w271, "Input--Potential"=w265, "Element"=T17."Square Wave") -> ("Output"=w264:T22, "Arduino Out"=w262:cluster{"Error Out":errorcluster, "LINX Out":T9})  [unwired: 5 in]
    }
    frame "Calibration" {
      w276 = 0.0
      n98 = Decrement(x="Cycles \n[Cal]") -> (x-1=w289:i32)
      n99 = Bundle("Ei (V)\n[Cal]"="Ei (V)\n[Cal]", w276, "E1 (V)\n[Cal]"="E1 (V)\n[Cal]", "E2 (V)\n[Cal]"="E2 (V)\n[Cal]", w276) -> (w290:T31)  [unwired: 1 in]
      n100 = Bundle(w276, "Resolution (ms)\n[Cal]"="Resolution (ms)\n[Cal]", w276, w289) -> (w288:T32)  [unwired: 1 in]
      n101 = Bundle("Scan Rate (V/s)\n[Cal]"="Scan Rate (V/s)\n[Cal]", 1.0) -> (w286:cluster{"Scan Rate (V/s)\n[Cal]":dbl, dbl})  [unwired: 1 in]
      n102 = call "Method Elements.vi"("Arduino In"=w280, "Potential Calibration"=w274, "Input--Scan Rate"=w286, "Input--Timing"=w288, "Input--Potential"=w290, "Element"=T17."Triangle Wave") -> ("Output"=w278:T22, "Arduino Out"=w279:cluster{"Error Out":errorcluster, "LINX Out":T9})  [unwired: 4 in]
    }
    frame "Method Builder" {
      # "no signal averaging... yet"
      n103 = call "Method Builder.vi"("Input A"="Input A", "Mode"="Mode", "Potential Calibration"=w292, "Input B"="Input B", "Input C"="Input C", "Input D"="Input D", "Input E"="Input E", "Cycles"="Cycles\n[MB]", "Arduino In"=w296) -> ("Output"=w294:T22, "Preview (Single Cycle)"=→"Preview (Single Cycle)":cluster{dbl[], "Preview":dbl[]}[], "Arduino Out"=w295:cluster{"Error Out":errorcluster, "LINX Out":T9}, "Signal Frequencies (mHz)"=→"Signal Frequencies (mHz)":cluster{"A":dbl, "B":dbl})  [unwired: 3 in]
    }
    frame "Analysis" {
    }
  }
  n104 = Build Array("Potential Calibration", "Current Calibration") -> (w12:dbl[][][])
  n105 = Unbundle By Name(w11) -> ("Wait Time (ms)"=w41:dbl, "Array Size"=w40:i32)
  n106 = case shown="\"Galvanostatic Cycling\"" "Method Selector" {
    tunnel: [w312 w323 w334 w345 w356 w367 w378 w389 w400 w411 path "" ("File Name Out")] -> w56
    tunnel: [w311 w322 w333 w344 w355 w366 w377 w388 w399 w410 FALSE ("Cancel Out")] -> w45
    tunnel: w22 -> [w310 w321 w332 w343 w354 w365 w376 w387 w398 w409 w421]
    tunnel: [w309 w320 w331 w342 w353 w364 w375 w386 w397 w408 w421] -> w21
    frame "OCP", Default {
      n107 = event shown="[1] \"Start\": Mouse Move;  \"Start\": Mouse Down;  \"Start\": Mouse Leave;  \"Start\": Mouse Up" {
        selector: _ -> [_ _]
        dyn-events: _ -> [_ _]
        timeout: 0 -> [_ _]
        tunnel: [TRUE ("Cancel Out") w319] -> w311
        tunnel: [path "" ("File Name Out") w318] -> w312
        tunnel: w310 -> [w314 w317]
        tunnel: [w314 w317] -> w309
        event Timeout {
          n108 = event-data() -> ()  [unwired: 1 in, 3 out]
        }
        event "Start": Mouse Move; "Start": Mouse Down; "Start": Mouse Leave; "Start": Mouse Up {
          n109 = event-data() -> ()  [unwired: 1 in, 3 out]
          n110 = call "File Dialog.vi"() -> ("Cancel Out"=w319:bool, "File Name Out"=w318:path)  [unwired: 10 in]
        }
      }
    }
    frame "CV" {
      n111 = event shown="[1] \"Start\": Mouse Move;  \"Start\": Mouse Down;  \"Start\": Mouse Leave;  \"Start\": Mouse Up" {
        selector: _ -> [_ _]
        dyn-events: _ -> [_ _]
        timeout: 0 -> [_ _]
        tunnel: [TRUE ("Cancel Out") w330] -> w322
        tunnel: [path "" ("File Name Out") w329] -> w323
        tunnel: w321 -> [w325 w328]
        tunnel: [w325 w328] -> w320
        event Timeout {
          n112 = event-data() -> ()  [unwired: 1 in, 3 out]
        }
        event "Start": Mouse Move; "Start": Mouse Down; "Start": Mouse Leave; "Start": Mouse Up {
          n113 = event-data() -> ()  [unwired: 1 in, 3 out]
          n114 = call "File Dialog.vi"() -> ("Cancel Out"=w330:bool, "File Name Out"=w329:path)  [unwired: 10 in]
        }
      }
    }
    frame "LSV" {
      n115 = event shown="[1] \"Start\": Mouse Move;  \"Start\": Mouse Down;  \"Start\": Mouse Leave;  \"Start\": Mouse Up" {
        selector: _ -> [_ _]
        dyn-events: _ -> [_ _]
        timeout: 0 -> [_ _]
        tunnel: [TRUE ("Cancel Out") w341] -> w333
        tunnel: [path "" ("File Name Out") w340] -> w334
        tunnel: w332 -> [w336 w339]
        tunnel: [w336 w339] -> w331
        event Timeout {
          n116 = event-data() -> ()  [unwired: 1 in, 3 out]
        }
        event "Start": Mouse Move; "Start": Mouse Down; "Start": Mouse Leave; "Start": Mouse Up {
          n117 = event-data() -> ()  [unwired: 1 in, 3 out]
          n118 = call "File Dialog.vi"() -> ("Cancel Out"=w341:bool, "File Name Out"=w340:path)  [unwired: 10 in]
        }
      }
    }
    frame "ASV" {
      n119 = event shown="[1] \"Start\": Mouse Move;  \"Start\": Mouse Down;  \"Start\": Mouse Leave;  \"Start\": Mouse Up" {
        selector: _ -> [_ _]
        dyn-events: _ -> [_ _]
        timeout: 0 -> [_ _]
        tunnel: [TRUE ("Cancel Out") w352] -> w344
        tunnel: [path "" ("File Name Out") w351] -> w345
        tunnel: w343 -> [w347 w350]
        tunnel: [w347 w350] -> w342
        event Timeout {
          n120 = event-data() -> ()  [unwired: 1 in, 3 out]
        }
        event "Start": Mouse Move; "Start": Mouse Down; "Start": Mouse Leave; "Start": Mouse Up {
          n121 = event-data() -> ()  [unwired: 1 in, 3 out]
          n122 = call "File Dialog.vi"() -> ("Cancel Out"=w352:bool, "File Name Out"=w351:path)  [unwired: 10 in]
        }
      }
    }
    frame "CA" {
      n123 = event shown="[1] \"Start\": Mouse Move;  \"Start\": Mouse Down;  \"Start\": Mouse Leave;  \"Start\": Mouse Up" {
        selector: _ -> [_ _]
        dyn-events: _ -> [_ _]
        timeout: 0 -> [_ _]
        tunnel: [TRUE ("Cancel Out") w363] -> w355
        tunnel: [path "" ("File Name Out") w362] -> w356
        tunnel: w354 -> [w358 w361]
        tunnel: [w358 w361] -> w353
        event Timeout {
          n124 = event-data() -> ()  [unwired: 1 in, 3 out]
        }
        event "Start": Mouse Move; "Start": Mouse Down; "Start": Mouse Leave; "Start": Mouse Up {
          n125 = event-data() -> ()  [unwired: 1 in, 3 out]
          n126 = call "File Dialog.vi"() -> ("Cancel Out"=w363:bool, "File Name Out"=w362:path)  [unwired: 10 in]
        }
      }
    }
    frame "CP" {
      n127 = event shown="[1] \"Start\": Mouse Move;  \"Start\": Mouse Down;  \"Start\": Mouse Leave;  \"Start\": Mouse Up" {
        selector: _ -> [_ _]
        dyn-events: _ -> [_ _]
        timeout: 0 -> [_ _]
        tunnel: [TRUE ("Cancel Out") w374] -> w366
        tunnel: [path "" ("File Name Out") w373] -> w367
        tunnel: w365 -> [w369 w372]
        tunnel: [w369 w372] -> w364
        event Timeout {
          n128 = event-data() -> ()  [unwired: 1 in, 3 out]
        }
        event "Start": Mouse Move; "Start": Mouse Down; "Start": Mouse Leave; "Start": Mouse Up {
          n129 = event-data() -> ()  [unwired: 1 in, 3 out]
          n130 = call "File Dialog.vi"() -> ("Cancel Out"=w374:bool, "File Name Out"=w373:path)  [unwired: 10 in]
        }
      }
    }
    frame "Galvanostatic Cycling" {
      n131 = event shown="[1] \"Start\": Mouse Move;  \"Start\": Mouse Down;  \"Start\": Mouse Leave;  \"Start\": Mouse Up" {
        selector: _ -> [_ _]
        dyn-events: _ -> [_ _]
        timeout: 0 -> [_ _]
        tunnel: [TRUE ("Cancel Out") w385] -> w377
        tunnel: [path "" ("File Name Out") w384] -> w378
        tunnel: w376 -> [w380 w383]
        tunnel: [w380 w383] -> w375
        event Timeout {
          n132 = event-data() -> ()  [unwired: 1 in, 3 out]
        }
        event "Start": Mouse Move; "Start": Mouse Down; "Start": Mouse Leave; "Start": Mouse Up {
          n133 = event-data() -> ()  [unwired: 1 in, 3 out]
          n134 = call "File Dialog.vi"() -> ("Cancel Out"=w385:bool, "File Name Out"=w384:path)  [unwired: 10 in]
        }
      }
    }
    frame "Ohmic Drop" {
      n135 = event shown="[1] \"Start\": Mouse Move;  \"Start\": Mouse Down;  \"Start\": Mouse Leave;  \"Start\": Mouse Up" {
        selector: _ -> [_ _]
        dyn-events: _ -> [_ _]
        timeout: 0 -> [_ _]
        tunnel: [TRUE ("Cancel Out") w396] -> w388
        tunnel: [path "" ("File Name Out") w395] -> w389
        tunnel: w387 -> [w391 w394]
        tunnel: [w391 w394] -> w386
        event Timeout {
          n136 = event-data() -> ()  [unwired: 1 in, 3 out]
        }
        event "Start": Mouse Move; "Start": Mouse Down; "Start": Mouse Leave; "Start": Mouse Up {
          n137 = event-data() -> ()  [unwired: 1 in, 3 out]
          n138 = call "File Dialog.vi"() -> ("Cancel Out"=w396:bool, "File Name Out"=w395:path)  [unwired: 10 in]
        }
      }
    }
    frame "Calibration" {
      n139 = event shown="[1] \"Start\": Mouse Move;  \"Start\": Mouse Down;  \"Start\": Mouse Leave;  \"Start\": Mouse Up" {
        selector: _ -> [_ _]
        dyn-events: _ -> [_ _]
        timeout: 0 -> [_ _]
        tunnel: [TRUE ("Cancel Out") w407] -> w399
        tunnel: [path "" ("File Name Out") w406] -> w400
        tunnel: w398 -> [w402 w405]
        tunnel: [w402 w405] -> w397
        event Timeout {
          n140 = event-data() -> ()  [unwired: 1 in, 3 out]
        }
        event "Start": Mouse Move; "Start": Mouse Down; "Start": Mouse Leave; "Start": Mouse Up {
          n141 = event-data() -> ()  [unwired: 1 in, 3 out]
          n142 = call "File Dialog.vi"() -> ("Cancel Out"=w407:bool, "File Name Out"=w406:path)  [unwired: 10 in]
        }
      }
    }
    frame "Method Builder" {
      n143 = event shown="[1] \"Start\": Mouse Move;  \"Start\": Mouse Down;  \"Start\": Mouse Leave;  \"Start\": Mouse Up" {
        selector: _ -> [_ _]
        dyn-events: _ -> [_ _]
        timeout: 0 -> [_ _]
        tunnel: [TRUE ("Cancel Out") w418] -> w410
        tunnel: [path "" ("File Name Out") w417] -> w411
        tunnel: w409 -> [w413 w416]
        tunnel: [w413 w416] -> w408
        event Timeout {
          n144 = event-data() -> ()  [unwired: 1 in, 3 out]
        }
        event "Start": Mouse Move; "Start": Mouse Down; "Start": Mouse Leave; "Start": Mouse Up {
          n145 = event-data() -> ()  [unwired: 1 in, 3 out]
          n146 = call "File Dialog.vi"() -> ("Cancel Out"=w418:bool, "File Name Out"=w417:path)  [unwired: 10 in]
        }
      }
    }
    frame "Analysis" {
    }
  }
  n147 = To Double Precision Float(number=w40) -> (double precision float=w20:dbl)
  n148 = Multiply(x=w41, y=w20) -> (x*y=w39:dbl)
  n149 = Divide(x=w39, y=1000.0) -> (x/y=w1:dbl)
  n150 = Index Array(array="Current Calibration", index (col)=1 ("disabled index (col)")) -> (element=w33:dbl[])  [unwired: 1 in]
  n151 = Index Array(array="Current Calibration", index (col)=2 ("disabled index (col)")) -> (element=w16:dbl[])  [unwired: 1 in]
  n152 = property on="Progress" class="Slide (strict)"("Scale.Maximum"=w1) -> ()  [unwired: 2 in, 2 out]
  n153 = Build Path(base path="Save Path", name or relative path=w56) -> (appended path=w30:path)
  n154 = To Long Integer(number="Sensitivity (Jumper)") -> (32bit integer=w15:i32)
  n155 = Unbundle(w21) -> ("Error Out"=w27:errorcluster, "LINX Resource"=w23:T9)
  n156 = Index Array(array=w16, index=w15) -> (element=w9:dbl)
  n157 = Index Array(array=w33, index=w15) -> (element=w10:dbl)
  n158 = Index Array(array="Potential Calibration", index (row) #1=w7, index (col) #1=w7, index (row) #2=w7, index (col) #2=1 ("disabled index (col)")) -> (element #1=w5:dbl, element #2=w4:dbl)
  n159 = case shown="\"Galvanostatic Cycling\"" "Method Selector" {
    tunnel: [w423 w426 w432 w438 w444 w450 w456 w461 w464 w470 w475] -> w25
    tunnel: w27 -> [w423 w427 w433 w439 w445 w451 w457 w461 w465 w471 w475]
    tunnel: [w422 w425 w431 w437 w443 w449 w455 w460 w463 w469 w474] -> w24
    tunnel: w23 -> [w422 w424 w430 w436 w442 w448 w454 w460 w462 w468 w474]
    frame "OCP", Default {
    }
    frame "CV" {
      n160 = call-poly <vilib>:"PWM Set Duty Cycle.vi"("Error In"=w427, "Duty Cycle (0-1)"=1.0, "PWM Channel"=u8 6 ("DO Channel"), "LINX Resource"=w424) -> ("Error Out"=w426:errorcluster, "LINX Resource"=w425:T9)  [unwired: 6 in]
    }
    frame "LSV" {
      n161 = call-poly <vilib>:"PWM Set Duty Cycle.vi"("Error In"=w433, "Duty Cycle (0-1)"=1.0, "PWM Channel"=u8 6 ("DO Channel"), "LINX Resource"=w430) -> ("Error Out"=w432:errorcluster, "LINX Resource"=w431:T9)  [unwired: 6 in]
    }
    frame "ASV" {
      n162 = call-poly <vilib>:"PWM Set Duty Cycle.vi"("Error In"=w439, "Duty Cycle (0-1)"=1.0, "PWM Channel"=u8 6 ("DO Channel"), "LINX Resource"=w436) -> ("Error Out"=w438:errorcluster, "LINX Resource"=w437:T9)  [unwired: 6 in]
    }
    frame "CA" {
      n163 = call-poly <vilib>:"PWM Set Duty Cycle.vi"("Error In"=w445, "Duty Cycle (0-1)"=1.0, "PWM Channel"=u8 6 ("DO Channel"), "LINX Resource"=w442) -> ("Error Out"=w444:errorcluster, "LINX Resource"=w443:T9)  [unwired: 6 in]
    }
    frame "CP" {
      n164 = call-poly <vilib>:"PWM Set Duty Cycle.vi"("Error In"=w451, "Duty Cycle (0-1)"=1.0, "PWM Channel"=u8 6 ("DO Channel"), "LINX Resource"=w448) -> ("Error Out"=w450:errorcluster, "LINX Resource"=w449:T9)  [unwired: 6 in]
    }
    frame "Galvanostatic Cycling" {
      n165 = call-poly <vilib>:"PWM Set Duty Cycle.vi"("Error In"=w457, "Duty Cycle (0-1)"=1.0, "PWM Channel"=u8 6 ("DO Channel"), "LINX Resource"=w454) -> ("Error Out"=w456:errorcluster, "LINX Resource"=w455:T9)  [unwired: 6 in]
    }
    frame "Ohmic Drop" {
    }
    frame "Calibration" {
      n166 = call-poly <vilib>:"PWM Set Duty Cycle.vi"("Error In"=w465, "Duty Cycle (0-1)"=1.0, "PWM Channel"=u8 6 ("DO Channel"), "LINX Resource"=w462) -> ("Error Out"=w464:errorcluster, "LINX Resource"=w463:T9)  [unwired: 6 in]
    }
    frame "Method Builder" {
      n167 = call-poly <vilib>:"PWM Set Duty Cycle.vi"("Error In"=w471, "Duty Cycle (0-1)"=1.0, "PWM Channel"=u8 6 ("DO Channel"), "LINX Resource"=w468) -> ("Error Out"=w470:errorcluster, "LINX Resource"=w469:T9)  [unwired: 6 in]
    }
    frame "Analysis" {
    }
  }
  n168 = Index Array(array="Current Calibration", index (col)=3 ("disabled index (col)")) -> (element=w62:dbl[])  [unwired: 1 in]
  n169 = Index Array(array=w62, index=w15) -> (element=w57:dbl)
  n170 = Build Array(w5, w4, w10, w9) -> (w3:dbl[])
  n171 = Index Array(array="Current Calibration", index (col)=4 ("disabled index (col)")) -> (element=w59:dbl[])  [unwired: 1 in]
  n172 = Index Array(array=w59, index=w15) -> (element=w58:dbl)
  n173 = Bundle("Error Out"=w25, "LINX Resource"=w24) -> (w26:T15)  [unwired: 1 in]
  n174 = case shown="True" w45 {
    tunnel: [w476 w477] -> w64
    frame False {
      n175 = call <vilib>:"High Resolution Relative Seconds.vi"() -> ("relative seconds"=w476:dbl)
    }
    frame True {
      n176 = call <vilib>:"High Resolution Relative Seconds.vi"() -> ("relative seconds"=w477:dbl)
    }
  }
  n177 = while {
    tunnel: "Method Selector" -> [w511]
    tunnel: w45 -> [w489]
    tunnel: w64 -> [w509]
    tunnel: w11 -> [w484]
    shift-right: [w500] -> _
    shift-left: w29 -> [w499]
    tunnel: w3 -> [w496]
    shift-right: [w494] -> _
    shift-left: w29 -> [w493]
    tunnel: w28 -> [w492]
    shift-right: [w495] -> w37
    shift-left: w26 -> [w491]
    tunnel: [w485] -> w2
    tunnel: w1 -> [w479]
    i -> [w510]
    stop <- w490 stop-if-true
    n178 = Divide(x=w479, y=60.0) -> (x/y=→"max time (min)":dbl)
    n179 = Unbundle By Name(w484) -> ("Wait Time (ms)"=w498:dbl, "Array Size"=w497:i32)
    n180 = case shown="\"OCP\", Default" w511 {
      tunnel: [w536 w576 w619 w673 w704 w735 w764 w819 w898 w943 FALSE ("Stop condition")] -> w488
      tunnel: w510 -> [w528 w560 w601 w656 w695 w733 w769 w807 w907 w934 _]
      tunnel: w509 -> [w542 w583 w626 w680 w709 w759 w794 w816 w914 w949 _]
      tunnel: [w540 w582 w625 w679 w708 w758 w793 w815 w913 w948 0.0] -> w482
      tunnel: [0.001 w543 w586 w643 w694 w715 w774 w814 w886 w933 0.0] -> w501
      tunnel: w491 -> [w538 w574 w616 w670 w699 w751 w786 w802 w899 w940 w982]
      tunnel: [w537 w573 w615 w669 w698 w750 w785 w801 w895 w939 w980] -> w495
      tunnel: [w535 w564 w602 w657 w701 w753 w788 w803 w882 w941 w975] -> w500
      tunnel: w499 -> [w534 w575 w618 w672 w702 w754 w789 w804 w901 w942 w975]
      tunnel: w498 -> [w533 w578 w621 w675 w693 w719 w775 w809 w911 w946 _]
      tunnel: w497 -> [w532 w577 w620 w674 w705 w755 w790 w808 w910 w945 _]
      tunnel: w496 -> [w521 w549 w589 w646 w703 w713 w772 w805 w894 w944 _]
      tunnel: [w523 w566 w609 w663 w691 w749 w784 w800 w897 w928 w974] -> w494
      tunnel: w493 -> [w523 w567 w610 w664 w690 w748 w783 w799 w896 w927 w974]
      tunnel: w492 -> [_ w565 w608 w642 w689 w747 w782 w798 w893 w926 _]
      tunnel: [w522 w553 w596 w651 w684 w744 w780 w797 w883 w924 T33 {"Elapsed Time (s)"=[], "E (V)"=[], "i (mA)"=[], "Vr (V)"=[], "Eraw (V)"=[]} ("Acquisition")] -> w485
      tunnel: w484 -> [_ w554 w597 w652 w683 w714 w773 w796 w890 w923 _]
      frame "OCP", Default {
        # "no rest for OCP"
        n181 = Bundle("Wait Time (ms)"=w533, w528, "Array Size"=w532, u32 0) -> (w530:T34)  [unwired: 1 in]
        n182 = call "OCP.vi"("Data In"=w534, "Timing"=w530, "Arduino In"=w538) -> ("Data Out"=w535:dbl[][], "Aquisition"=w522:T33, "Stop condition"=w536:bool, "Arduino Out"=w537:cluster{"error out":errorcluster, "LINX out":T9})  [unwired: 3 in]
        n183 = call <vilib>:"High Resolution Relative Seconds.vi"() -> ("relative seconds"=w541:dbl)
        n184 = Unbundle By Name(w522) -> ("Elapsed Time (s)"=w529:dbl[], "E (V)"=w518:dbl[])
        n185 = Subtract(x=w541, y=w542) -> (x-y=w525:dbl)
        n186 = Decrement(x=w528) -> (x-1=w524:i32)
        n187 = Index Array(array=w521, index #1=1 ("index"), index #2=0 ("index")) -> (element #1=w516:dbl, element #2=w515:dbl)
        n188 = Multiply(x=w515, y=w518) -> (x*y=w517:dbl[])
        n189 = Absolute Value(x=w525) -> (abs(x)=w540:dbl)
        n190 = Add(x=w516, y=w517) -> (x+y=w514:dbl[])
        n191 = Bundle("Elapsed Time (s)"=w529, w514) -> (→"Open Circuit":cluster{"Elapsed Time (s)":dbl[], dbl[]})  [unwired: 1 in]
        n192 = Index Array(array=w514, index=w524) -> (element=→"OCP (V)":dbl)
      }
      frame "CV" {
        # "rest"
        # "2 s rest"
        n193 = Bundle("Wait Time (ms)"=w578, w560, "Array Size"=w577, u32 2000) -> (w572:T34)  [unwired: 1 in]
        n194 = call "Acquire.vi"("Correction and Conversion"=w549, "Timing"=w572, "Averaging and Conversion"=w565, "Method Output"=w554, "Data In"=w575, "Average In"=w567, "Calibration?"=FALSE, "Arduino In"=w574) -> ("Stop condition"=w576:bool, "Acquisition"=w553:T33, "Data Out"=w564:dbl[][], "Average Out"=w566:dbl[][], "Arduino Out"=w573:cluster{"error out":errorcluster, "LINX out":T9})  [unwired: 7 in]
        n195 = call <vilib>:"High Resolution Relative Seconds.vi"() -> ("relative seconds"=w585:dbl)
        n196 = Subtract(x=w585, y=w583) -> (x-y=w584:dbl)
        n197 = Unbundle By Name(w553) -> ("Elapsed Time (s)"=w552:dbl[], "E (V)"=w551:dbl[], "i (mA)"=w550:dbl[])
        n198 = Subtract(x=w584, y=2.0) -> (x-y=w581:dbl)
        n199 = Absolute Value(x=w581) -> (abs(x)=w582:dbl)
        n200 = Bundle("Elapsed Time (s)"=w552, "i (mA)"=w550) -> (w570:T35)  [unwired: 1 in]
        n201 = Bundle("Elapsed Time (s)"=w552, "E (V)"=w551) -> (w571:cluster{"Elapsed Time (s)":dbl[], "E (V)":dbl[]})  [unwired: 1 in]
        n202 = Decrement(x=w560) -> (x-1=w556:i32)
        n203 = Build Array(w571, w570) -> (→"Applied and Response (CV)":T2)
        n204 = Bundle("E (V)"=w551, "i (mA)"=w550) -> (→"Cyclic Voltammagram":cluster{"E (V)":dbl[], "i (mA)":dbl[]})  [unwired: 1 in]
        n205 = Index Array(array=w564, index (row)=w556, index (col)=3 ("disabled index (col)")) -> (element=w559:dbl)
        n206 = Index Array(array=w564, index (row)=w556, index (col)=1 ("disabled index (col)")) -> (element=→"E (V)\n[CV]":dbl)
        n207 = Index Array(array=w549, index #1=3 ("index"), index #2=2 ("index")) -> (element #1=w545:dbl, element #2=w544:dbl)
        n208 = Subtract(x=w559, y=2.5 ("x")) -> (x-y=w557:dbl)
        n209 = Multiply(x=w544, y=w557) -> (x*y=w547:dbl)
        n210 = Add(x=w545, y=w547) -> (x+y=w543:dbl)
        "i (mA)\n[CV]" <- w543
      }
      frame "LSV" {
        # "rest"
        # "3 s rest"
        n211 = Bundle("Wait Time (ms)"=w621, w601, "Array Size"=w620, u32 3000) -> (w617:T34)  [unwired: 1 in]
        n212 = call "Acquire.vi"("Correction and Conversion"=w589, "Timing"=w617, "Averaging and Conversion"=w608, "Method Output"=w597, "Data In"=w618, "Average In"=w610, "Calibration?"=FALSE, "Arduino In"=w616) -> ("Stop condition"=w619:bool, "Acquisition"=w596:T33, "Data Out"=w602:dbl[][], "Average Out"=w609:dbl[][], "Arduino Out"=w615:cluster{"error out":errorcluster, "LINX out":T9})  [unwired: 7 in]
        n213 = call <vilib>:"High Resolution Relative Seconds.vi"() -> ("relative seconds"=w628:dbl)
        n214 = Unbundle By Name(w596) -> ("Elapsed Time (s)"=w595:dbl[], "E (V)"=w594:dbl[], "i (mA)"=w593:dbl[])
        n215 = Subtract(x=w628, y=w626) -> (x-y=w627:dbl)
        n216 = Bundle("E (V)"=w594, "i (mA)"=w593) -> (→"Linear Sweep Voltammagram":cluster{"E (V)":dbl[], "i (mA)":dbl[]})  [unwired: 1 in]
        n217 = Bundle("Elapsed Time (s)"=w595, "E (V)"=w594) -> (w614:cluster{"Elapsed Time (s)":dbl[], "E (V)":dbl[]})  [unwired: 1 in]
        n218 = Bundle("Elapsed Time (s)"=w595, "i (mA)"=w593) -> (w613:T35)  [unwired: 1 in]
        n219 = Subtract(x=w627, y=3.0) -> (x-y=w624:dbl)
        n220 = Build Array(w614, w613) -> (→"Applied and Response (LSV)":T2)
        n221 = Decrement(x=w601) -> (x-1=w600:i32)
        n222 = Absolute Value(x=w624) -> (abs(x)=w625:dbl)
        n223 = Index Array(array=w602, index (row)=w600, index (col)=3 ("disabled index (col)")) -> (element=w605:dbl)
        n224 = Index Array(array=w602, index (row)=w600, index (col)=1 ("disabled index (col)")) -> (element=→"E (V)\n[lsv]":dbl)
        n225 = Index Array(array=w589, index #1=3 ("index"), index #2=2 ("index")) -> (element #1=w587:dbl, element #2=w588:dbl)
        n226 = Subtract(x=w605, y=2.5 ("x")) -> (x-y=w603:dbl)
        n227 = Multiply(x=w588, y=w603) -> (x*y=w590:dbl)
        n228 = Add(x=w587, y=w590) -> (x+y=w586:dbl)
        "i (mA)\n[LSV]" <- w586
      }
      frame "ASV" {
        w629 = 0 ("index")
        # "removes data associated with cleaning/ deposition"
        # "rest"
        # "3 s rest"
        n229 = Bundle("Wait Time (ms)"=w675, w656, "Array Size"=w674, u32 3000) -> (w671:T34)  [unwired: 1 in]
        n230 = Unbundle By Name(w642) -> ("Step Width"=w634:dbl)
        n231 = call "Acquire.vi"("Correction and Conversion"=w646, "Timing"=w671, "Averaging and Conversion"=w642, "Method Output"=w652, "Data In"=w672, "Average In"=w664, "Calibration?"=FALSE, "Arduino In"=w670) -> ("Stop condition"=w673:bool, "Acquisition"=w651:T33, "Data Out"=w657:dbl[][], "Average Out"=w663:dbl[][], "Arduino Out"=w669:cluster{"error out":errorcluster, "LINX out":T9})  [unwired: 7 in]
        n232 = local read "Time (s)\n(cleaning)"() -> (w639:dbl)
        n233 = local read "Time (s)\n(dep)"() -> (w638:dbl)
        n234 = call <vilib>:"High Resolution Relative Seconds.vi"() -> ("relative seconds"=w682:dbl)
        n235 = Unbundle By Name(w651) -> ("Elapsed Time (s)"=w650:dbl[], "E (V)"=w632:dbl[], "i (mA)"=w641:dbl[])
        n236 = Subtract(x=w682, y=w680) -> (x-y=w681:dbl)
        n237 = Add(x=w639, y=w638) -> (x+y=w637:dbl)
        n238 = Divide(x=w637, y=0.02) -> (x/y=w635:dbl)
        n239 = Divide(x=w635, y=w634) -> (x/y=w633:dbl)
        n240 = Bundle("Elapsed Time (s)"=w650, "E (V)"=w632) -> (w668:cluster{"Elapsed Time (s)":dbl[], "E (V)":dbl[]})  [unwired: 1 in]
        n241 = Bundle("Elapsed Time (s)"=w650, "i (mA)"=w641) -> (w667:T35)  [unwired: 1 in]
        n242 = To Long Integer(number=w633) -> (32bit integer=w630:i32)
        n243 = Subtract(x=w681, y=3.0) -> (x-y=w678:dbl)
        n244 = Build Array(w668, w667) -> (→"Applied and Response (ASV)":T2)
        n245 = Delete From Array(array=w641, length=w630, index=w629) -> (array with subset deleted=w640:dbl[])  [unwired: 1 out]
        n246 = Delete From Array(array=w632, length=w630, index=w629) -> (array with subset deleted=w631:dbl[])  [unwired: 1 out]
        n247 = Decrement(x=w656) -> (x-1=w655:i32)
        n248 = Bundle("E (V)"=w631, "i (mA)"=w640) -> (→"Anodic Stripping\n Voltammagram":cluster{"E (V)":dbl[], "i (mA)":dbl[]})  [unwired: 1 in]
        n249 = Absolute Value(x=w678) -> (abs(x)=w679:dbl)
        n250 = Index Array(array=w657, index (row)=w655, index (col)=3 ("disabled index (col)")) -> (element=w660:dbl)
        n251 = Index Array(array=w657, index (row)=w655, index (col)=1 ("disabled index (col)")) -> (element=→"E (V)\n[ASV]":dbl)
        n252 = Index Array(array=w646, index #1=3 ("index"), index #2=2 ("index")) -> (element #1=w644:dbl, element #2=w645:dbl)
        n253 = Subtract(x=w660, y=2.5 ("x")) -> (x-y=w658:dbl)
        n254 = Multiply(x=w645, y=w658) -> (x*y=w647:dbl)
        n255 = Add(x=w644, y=w647) -> (x+y=w643:dbl)
        "i (mA)\n[ASV]" <- w643
      }
      frame "CA" {
        # "no rest"
        n256 = Bundle("Wait Time (ms)"=w693, w695, "Array Size"=w705, u32 0) -> (w700:T34)  [unwired: 1 in]
        n257 = call "Acquire.vi"("Correction and Conversion"=w703, "Timing"=w700, "Averaging and Conversion"=w689, "Method Output"=w683, "Data In"=w702, "Average In"=w690, "Calibration?"=FALSE, "Arduino In"=w699) -> ("Stop condition"=w704:bool, "Acquisition"=w684:T33, "Data Out"=w701:dbl[][], "Average Out"=w691:dbl[][], "Arduino Out"=w698:cluster{"error out":errorcluster, "LINX out":T9})  [unwired: 7 in]
        n258 = call <vilib>:"High Resolution Relative Seconds.vi"() -> ("relative seconds"=w710:dbl)
        n259 = Subtract(x=w710, y=w709) -> (x-y=w707:dbl)
        n260 = Unbundle By Name(w684) -> ("Elapsed Time (s)"=w697:dbl[], "i (mA)"=w692:dbl[])
        n261 = Decrement(x=w695) -> (x-1=w688:i32)
        n262 = Absolute Value(x=w707) -> (abs(x)=w708:dbl)
        n263 = Index Array(array=w692, index=w688) -> (element=w694:dbl)
        "i (mA)\n[CA]" <- w694
        n264 = call <vilib>:"Integral x(t).vi"("dt"=w693, "X"=w692) -> ("Integral X"=w712:dbl[])  [unwired: 8 in, 1 out]
        n265 = Bundle("Elapsed Time (s)"=w697, "i (mA)"=w692) -> (→"Chronoamperometry":T35)  [unwired: 1 in]
        n266 = Index Array(array=w712, index=w688) -> (element=w711:dbl)
        n267 = Divide(x=w711, y=1000000.0) -> (x/y=→"q (C)":dbl)
      }
      frame "CP" {
        # "Energy = V(q)*dq\nmJ = V*(ms*mA/1000000)"
        # "end adquisition if Eapp falls below threshold"
        # "no rest"
        n268 = Bundle("Wait Time (ms)"=w719, w733, "Array Size"=w755, u32 0) -> (w752:T34)  [unwired: 1 in]
        n269 = Less?(x=w733, y=4) -> (x < y?=w731:bool)
        n270 = call "Acquire.vi"("Correction and Conversion"=w713, "Timing"=w752, "Averaging and Conversion"=w747, "Method Output"=w714, "Data In"=w754, "Average In"=w748, "Calibration?"=TRUE, "Arduino In"=w751) -> ("Stop condition"=w734:bool, "Acquisition"=w744:T33, "Data Out"=w753:dbl[][], "Average Out"=w749:dbl[][], "Arduino Out"=w750:cluster{"error out":errorcluster, "LINX out":T9})  [unwired: 7 in]
        n271 = Unbundle By Name(w744) -> ("Elapsed Time (s)"=w741:dbl[], "Eraw (V)"=w723:dbl[])
        n272 = call <vilib>:"High Resolution Relative Seconds.vi"() -> ("relative seconds"=w760:dbl)
        n273 = local read "Set Current (mA)\n[CP]"() -> (w715:dbl)
        n274 = Subtract(x=w760, y=w759) -> (x-y=w757:dbl)
        n275 = Decrement(x=w733) -> (x-1=w721:i32)
        n276 = Absolute Value(x=w757) -> (abs(x)=w758:dbl)
        n277 = Index Array(array=w741, index=w721) -> (element=w740:dbl)
        n278 = Index Array(array=w723, index=w721) -> (element=w725:dbl)
        "E (V)\n[CP]" <- w725
        n279 = Bundle("Elapsed Time (s)"=w741, "Eraw (V)"=w723) -> (→"Chronopotentiometry":T36)  [unwired: 1 in]
        n280 = Less Than 0?(x=w715) -> (x < 0?=w739:bool)
        n281 = call <vilib>:"Integral x(t).vi"("dt"=w719, "X"=w723) -> ("Integral X"=w722:dbl[])  [unwired: 8 in, 1 out]
        n282 = Greater Or Equal?(x=w725, y="Potential (V)\n[CP]") -> (x >= y?=w738:bool)
        n283 = Less Or Equal?(x=w725, y="Potential (V)\n[CP]") -> (x <= y?=w737:bool)
        n284 = Multiply(x=w715, y=w740) -> (x*y=w742:dbl)
        n285 = Multiply(x=w725, y=w715) -> (x*y=w727:dbl)
        n286 = Divide(x=w742, y=1000.0) -> (x/y=→"q (C)\n[CP]":dbl)
        n287 = Index Array(array=w722, index=w721) -> (element=w716:dbl)
        n288 = Select(t=w738, s=w739, f=w737) -> (s? t:f=w728:bool)
        n289 = Select(t=FALSE, s=w731, f=w728) -> (s? t:f=w729:bool)
        n290 = Or(x=w729, y=w734) -> (x .or. y?=w735:bool)
        n291 = Absolute Value(x=w727) -> (abs(x)=→"P (mW)\n[CP]":dbl)
        n292 = Compound Arithmetic op=MULTIPLY(w716, w715, 1e-06 ("value")) -> (w717:dbl)
        n293 = Absolute Value(x=w717) -> (abs(x)=→"Energy Delivered (J)\n[CP]":dbl)
      }
      frame "Galvanostatic Cycling" {
        # "no rest"
        n294 = Bundle("Wait Time (ms)"=w775, w769, "Array Size"=w790, u32 0) -> (w787:T34)  [unwired: 1 in]
        n295 = Less?(x=w769, y=4) -> (x < y?=w761:bool)
        n296 = call "Acquire.vi"("Correction and Conversion"=w772, "Timing"=w787, "Averaging and Conversion"=w782, "Method Output"=w773, "Data In"=w789, "Average In"=w783, "Calibration?"=TRUE, "Arduino In"=w786) -> ("Stop condition"=w763:bool, "Acquisition"=w780:T33, "Data Out"=w788:dbl[][], "Average Out"=w784:dbl[][], "Arduino Out"=w785:cluster{"error out":errorcluster, "LINX out":T9})  [unwired: 7 in]
        n297 = Unbundle By Name(w780) -> ("Elapsed Time (s)"=w779:dbl[], "Eraw (V)"=w777:dbl[])
        n298 = call <vilib>:"High Resolution Relative Seconds.vi"() -> ("relative seconds"=w795:dbl)
        n299 = local read "Set Current (mA)\n[CP]"() -> (w774:dbl)
        n300 = Subtract(x=w795, y=w794) -> (x-y=w792:dbl)
        n301 = Decrement(x=w769) -> (x-1=w776:i32)
        n302 = Absolute Value(x=w792) -> (abs(x)=w793:dbl)
        n303 = Index Array(array=w779, index=w776) -> (element=w778:dbl)
        n304 = Index Array(array=w777, index=w776) -> (element=w765:dbl)
        "E (V)\n[GC]" <- w765
        n305 = Less Or Equal?(x=w765, y=0.0) -> (x <= y?=w767:bool)
        n306 = Select(t=FALSE, s=w761, f=w767) -> (s? t:f=w762:bool)
        n307 = Or(x=w762, y=w763) -> (x .or. y?=w764:bool)
        n308 = Bundle("Elapsed Time (s)"=w779, "Eraw (V)"=w777) -> (→"Galvanostatic Cycling":T36)  [unwired: 1 in]
        n309 = Multiply(x=w774, y=w778) -> ()  [unwired: 1 out]
      }
      frame "Ohmic Drop" {
        # "0.2 s rest"
        # "rest"
        n310 = Bundle("Wait Time (ms)"=w809, w807, "Array Size"=w808, u32 200) -> (w806:T34)  [unwired: 1 in]
        n311 = case shown="True" "Measure Ru" {
          tunnel: [w834 w866] -> w819
          tunnel: [0.0 w854] -> w814
          tunnel: w806 -> [_ w859]
          tunnel: w805 -> [_ w867]
          tunnel: w804 -> [w824 w865]
          tunnel: [w824 w864] -> w803
          tunnel: w802 -> [w823 w846]
          tunnel: [w822 w863] -> w801
          tunnel: [T33 {"Elapsed Time (s)"=[], "E (V)"=[], "i (mA)"=[], "Vr (V)"=[], "Eraw (V)"=[]} ("Acquisition") w852] -> w797
          tunnel: [w821 w850] -> w800
          tunnel: w799 -> [w821 w849]
          tunnel: w798 -> [_ w848]
          tunnel: w796 -> [_ w835]
          frame False {
            n312 = control-ref of="Current Calibration"() -> (w831:refnum<vi>)
            n313 = local read "Measure Ru"() -> (w834:bool)
            n314 = control-ref of="Sensitivity (Jumper)"() -> (w832:refnum<vi>)
            n315 = call "Measure Ru.vi"("Arduino In"=w823, "reference in"=w831, "Ring in"=w832) -> ("Arduino Out"=w822:T37, "Ru"=w830:dbl)  [unwired: 5 in, 2 out]
            "Ru (Ohm)" <- w830
            n316 = Divide(x="% Compensation", y=100.0) -> (x/y=w828:dbl)
            n317 = Multiply(x=w830, y=w828) -> (x*y=→"Rc (Ohm)":dbl)
            n318 = Wait (ms)(milliseconds to wait=u32 500) -> ()  [unwired: 1 out]
          }
          frame True {
            # "turns off d3 after measuring Ru"
            n319 = Unbundle(w846) -> ("Error Out"=w845:errorcluster, "LINX Resource"=w844:T9)
            n320 = Unbundle(w859) -> (w856:i32)  [unwired: 3 out]
            n321 = call-poly <vilib>:"Digital Read.vi"("Error In"=w845, "DI Channel"=u8 3, "LINX Resource"=w844) -> ("Error Out"=w837:errorcluster, "LINX Resource"=w840:T9)  [unwired: 6 in, 1 out]
            n322 = Decrement(x=w856) -> (x-1=w851:i32)
            n323 = call-poly <vilib>:"PWM Set Duty Cycle.vi"("Error In"=w837, "Duty Cycle (0-1)"=1.0, "PWM Channel"=u8 6 ("DO Channel"), "LINX Resource"=w840) -> ("Error Out"=w838:errorcluster, "LINX Resource"=w839:T9)  [unwired: 6 in]
            n324 = Bundle("Error Out"=w838, "LINX Resource"=w839) -> (w836:T15)  [unwired: 1 in]
            n325 = call "Acquire.vi"("Correction and Conversion"=w867, "Timing"=w859, "Averaging and Conversion"=w848, "Method Output"=w835, "Data In"=w865, "Average In"=w849, "Calibration?"=TRUE, "Arduino In"=w836) -> ("Stop condition"=w866:bool, "Acquisition"=w852:T33, "Data Out"=w864:dbl[][], "Average Out"=w850:dbl[][], "Arduino Out"=w863:cluster{"error out":errorcluster, "LINX out":T9})  [unwired: 7 in]
            n326 = Unbundle By Name(w852) -> ("Elapsed Time (s)"=w862:dbl[], "Eraw (V)"=w855:dbl[], "i (mA)"=w858:dbl[])
            n327 = Index Array(array=w858, index=w851) -> (element=w854:dbl)
            "i (mA)\n[iR]" <- w854
            n328 = Bundle("Elapsed Time (s)"=w862, "Eraw (V)"=w855) -> (w861:T36)  [unwired: 1 in]
            n329 = Bundle("Elapsed Time (s)"=w862, "i (mA)"=w858) -> (w860:T35)  [unwired: 1 in]
            n330 = Index Array(array=w855, index=w851) -> (element=→"Eap (V)\n[iR]":dbl)
            n331 = Build Array(w861, w860) -> (→"Applied and Response (Ohmic)":T2)
          }
        }
        n332 = call <vilib>:"High Resolution Relative Seconds.vi"() -> ("relative seconds"=w817:dbl)
        n333 = Subtract(x=w817, y=w816) -> (x-y=w812:dbl)
        n334 = Subtract(x=w812, y=0.2) -> (x-y=w813:dbl)
        n335 = Absolute Value(x=w813) -> (abs(x)=w815:dbl)
      }
      frame "Calibration" {
        # "Vr = Em + b\nE = (Vr - b)/m\n\nOhm's law:\nE = iR, hence:\n\niR = (Vr - b)/m\ni = (Vr - b)/(mR) or\n\ni = Vr/mR - b/mR:\n1/mR = A/V conversion\n1000/mR = mA/V conversion\nand\n-1000b/mR = i offset (in mA)"
        # "rest"
        # "2 s rest"
        n336 = Bundle("Wait Time (ms)"=w911, w907, "Array Size"=w910, u32 2000) -> (w900:T34)  [unwired: 1 in]
        n337 = call "Acquire.vi"("Correction and Conversion"=w894, "Timing"=w900, "Averaging and Conversion"=w893, "Method Output"=w890, "Data In"=w901, "Average In"=w896, "Calibration?"=TRUE, "Arduino In"=w899) -> ("Stop condition"=w898:bool, "Acquisition"=w883:T33, "Data Out"=w882:dbl[][], "Average Out"=w897:dbl[][], "Arduino Out"=w895:cluster{"error out":errorcluster, "LINX out":T9})  [unwired: 7 in]
        n338 = Unbundle By Name(w883) -> ("E (V)"=w878:dbl[], "Eraw (V)"=w873:dbl[])
        n339 = Unbundle By Name(w883) -> ("Vr (V)"=w884:dbl[], "Eraw (V)"=w885:dbl[])
        n340 = Unbundle By Name(w883) -> ("Elapsed Time (s)"=w889:dbl[], "Eraw (V)"=w888:dbl[], "i (mA)"=w887:dbl[])
        n341 = call <vilib>:"High Resolution Relative Seconds.vi"() -> ("relative seconds"=w918:dbl)
        n342 = Subtract(x=w918, y=w914) -> (x-y=w917:dbl)
        n343 = Divide(x=1000.0, y="Sample Cell  Resistance (Ohm)") -> (x/y=w921:dbl)
        n344 = Decrement(x=w907) -> (x-1=w891:i32)
        n345 = call <vilib>:"Linear Fit.vi"("Y"=w884, "X"=w885) -> ("Best Linear Fit"=w903:dbl[], "slope"=w919:dbl, "intercept"=w870:dbl)  [unwired: 9 in, 2 out]
        n346 = call <vilib>:"Linear Fit.vi"("Y"=w873, "X"=w878) -> ("Best Linear Fit"=w875:dbl[], "slope"=→"E Conversion":dbl, "intercept"=→"E Offset\n[Cal]":dbl)  [unwired: 9 in, 2 out]
        n347 = Subtract(x=w917, y=2.0) -> (x-y=w915:dbl)
        n348 = Bundle("Elapsed Time (s)"=w889, "Eraw (V)"=w888) -> (w909:T36)  [unwired: 1 in]
        n349 = Bundle("Elapsed Time (s)"=w889, "i (mA)"=w887) -> (w906:T35)  [unwired: 1 in]
        n350 = Index Array(array=w887, index=w891) -> (element=w886:dbl)
        n351 = Bundle("E (V)"=w878, "Eraw (V)"=w873) -> (w881:cluster{"E (V)":dbl[], "Eraw (V)":dbl[]})  [unwired: 1 in]
        n352 = Bundle("E (V)"=w878, "Best Linear Fit"=w875) -> (w880:cluster{"E (V)":dbl[], "Best Linear Fit":dbl[]})  [unwired: 1 in]
        n353 = Divide(x=w921, y=w919) -> (x/y=w869:dbl)
        "i Conversion" <- w869
        n354 = Absolute Value(x=w915) -> (abs(x)=w913:dbl)
        n355 = Bundle("Eraw (V)"=w885, "Vr (V)"=w884) -> (w905:cluster{"Eraw (V)":dbl[], "Vr (V)":dbl[]})  [unwired: 1 in]
        n356 = call <vilib>:"Goodness of Fit.vi"("Best Fit"=w903, "Y"=w884) -> ("R-square"=→"R²\n[Calib] i":dbl)  [unwired: 6 in, 3 out]
        n357 = Build Array(w909, w906) -> (→"Applied and Response (Cal)":T2)
        n358 = Build Array(w881, w880) -> (→"E Calibration":T38)
        n359 = Bundle("Eraw (V)"=w885, "Best Linear Fit"=w903) -> (w902:T39)  [unwired: 1 in]
        n360 = Build Array(w905, w902) -> (→"i Calibration":T40)
        n361 = Compound Arithmetic op=MULTIPLY(w870, w869, -1.0 ("value")) -> (→"i Offset\n[Cal]":dbl)
        n362 = call <vilib>:"Goodness of Fit.vi"("Best Fit"=w875, "Y"=w873) -> ("R-square"=→"R²\n[Calib] E":dbl)  [unwired: 6 in, 3 out]
      }
      frame "Method Builder" {
        # "rest"
        # "2 s rest"
        n363 = Bundle("Wait Time (ms)"=w946, w934, "Array Size"=w945, u32 2000) -> (w938:T34)  [unwired: 1 in]
        n364 = call "Acquire.vi"("Correction and Conversion"=w944, "Timing"=w938, "Averaging and Conversion"=w926, "Method Output"=w923, "Data In"=w942, "Average In"=w927, "Calibration?"=FALSE, "Arduino In"=w940) -> ("Stop condition"=w943:bool, "Acquisition"=w924:T33, "Data Out"=w941:dbl[][], "Average Out"=w928:dbl[][], "Arduino Out"=w939:cluster{"error out":errorcluster, "LINX out":T9})  [unwired: 7 in]
        n365 = call <vilib>:"High Resolution Relative Seconds.vi"() -> ("relative seconds"=w953:dbl)
        n366 = Unbundle By Name(w924) -> ("Elapsed Time (s)"=w936:dbl[], "i (mA)"=w930:dbl[], "E (V)"=w931:dbl[])
        n367 = Subtract(x=w953, y=w949) -> (x-y=w951:dbl)
        n368 = Decrement(x=w934) -> (x-1=w932:i32)
        n369 = Subtract(x=w951, y=2.0) -> (x-y=w952:dbl)
        n370 = Absolute Value(x=w952) -> (abs(x)=w948:dbl)
        n371 = Bundle("Elapsed Time (s)"=w936, "i (mA)"=w930) -> (→"Method i-t":T35)  [unwired: 1 in]
        n372 = Bundle("E (V)"=w931, "i (mA)"=w930) -> (→"Method i-E":cluster{"E (V)":dbl[], "i (mA)":dbl[]})  [unwired: 1 in]
        n373 = Index Array(array=w930, index=w932) -> (element=w933:dbl)
        "i (mA)\n[MB]" <- w933
        n374 = Index Array(array=w931, index=w932) -> (element=→"E (V)\nMB":dbl)
      }
      frame "Analysis" {
        # "Cycle selector"
        n375 = Unbundle(w982) -> ("Error Out"=w989:errorcluster, "LINX Resource"=w979:T9)
        n376 = call-poly <vilib>:"Read Delimited Spreadsheet.vi"("file path (dialog if empty)"="Open Data", "error in (no error)"=w989, "transpose? (F)"=TRUE, "delimiter (\\t)"="," ("delimiter (\\t)")) -> ("all rows"=w990:dbl[][], "error out"=w970:errorcluster)  [unwired: 6 in, 4 out]
        n377 = Increment(x="Cycle") -> (x+1=w955:dbl)
        n378 = Delete From Array(array=w990, length=2, index (col)=0 ("disabled index (col)")) -> (array with subset deleted=w962:dbl[][])  [unwired: 1 in, 1 out]
        n379 = Index Array(array=w962, index (row)=2) -> (element=w960:dbl[])  [unwired: 1 in]
        n380 = Array Max & Min(array=w960) -> (max value=w959:dbl)  [unwired: 3 out]
        n381 = To Long Integer(number=w959) -> (32bit integer=w958:i32)
        n382 = Search 1D Array(1D array=w960, element=2.0) -> (index of element=w963:i32)  [unwired: 1 in]
        n383 = for {
          N: w958 -> [_]
          shift-right: [w997] -> w957
          shift-left: string[] [] ("Strings []") -> [w996]
          i -> [w995]
          n384 = Increment(x=w995) -> (x+1=w993:i32)
          n385 = Number To Decimal String(number=w993) -> (decimal integer string=w994:string)  [unwired: 1 in]
          n386 = Insert Into Array(array=w996, new element=w994) -> (w997:string[])  [unwired: 1 in]
        }
        n387 = Equal?(x=w963, y=-1) -> (x = y?=w964:bool)
        n388 = case shown="False" w964 {
          tunnel: w962 -> [w998 w1004]
          tunnel: [w998 w1003] -> w967
          tunnel: w963 -> [_ w1002]
          tunnel: w960 -> [_ w1001]
          tunnel: w955 -> [_ w1000]
          frame True {
          }
          frame False {
            n389 = Search 1D Array(1D array=w1001, element=w1000) -> (index of element=w999:i32)  [unwired: 1 in]
            n390 = Array Subset(array=w1004, index (col)=w999, length (col)=w1002) -> (w1003:dbl[][])  [unwired: 2 in]
          }
        }
        n391 = Index Array(array=w967, index (row) #1=0 ("index (row)"), index (row) #2=1 ("index (row)")) -> (element #1=w991:dbl[], element #2=w992:dbl[])  [unwired: 2 in]
        n392 = property on="Cycle" class="Ring (strict)"("Strings []"=w957) -> ()  [unwired: 2 in, 2 out]
        n393 = Bundle("all rows"=w991, "all rows"=w992) -> (w972:cluster{"all rows":dbl[], "all rows":dbl[]})  [unwired: 1 in]
        n394 = case shown="1" "Plot Type" {
          tunnel: w972 -> [w1015 w1035]
          tunnel: [w1014 w1034] -> w971
          tunnel: w970 -> [w1006 w1033]
          tunnel: [w1005 w1032] -> w969
          frame 0, Default {
            n395 = Build Array(w1015, cluster{"all rows":dbl[], "all rows":dbl[]} {"all rows"=[], "all rows"=[]} ("element")) -> (w1014:cluster{"all rows":dbl[], "all rows":dbl[]}[])
            n396 = property on="Analysis" class="XYGraph (strict)"(error in=w1006, "Active Cursor"=u32 0, "Cursor.Visible"=TRUE, "Active Cursor"=u32 1, "Cursor.Visible"=TRUE, "XScale.NameLbl.Text"="E (V vs ref)" ("X Scale.Name Label.Text"), "YScale.NameLbl.Text"="i (mA)" ("Y Scale.Name Label.Text")) -> (error out=w1005:errorcluster)  [unwired: 1 in, 1 out]
          }
          frame 1 {
            n397 = Unbundle(w1035) -> ("all rows"=w1049:dbl[], "all rows"=w1047:dbl[])
            n398 = Absolute Value(x=w1047) -> (abs(x)=w1046:dbl[])
            n399 = Logarithm Base 10(1:w1046) -> (0:w1020:dbl[])
            n400 = property on="Analysis" class="XYGraph (strict)"(error in=w1033, "Active Cursor"=u32 0, "Cursor.Visible"=TRUE, "Active Cursor"=u32 1, "Cursor.Visible"=TRUE, "XScale.NameLbl.Text"="log |i/mA|" ("X Scale.Name Label.Text"), "YScale.NameLbl.Text"="E - E0 (V)" ("Y Scale.Name Label.Text")) -> (error out=w1032:errorcluster, "Cursor.Cursor Index"=w1026:i32, "Cursor.Cursor Index"=w1027:i32)  [unwired: 1 in, 1 out]
            n401 = Subtract(x=w1027, y=w1026) -> (x-y=w1044:i32)
            n402 = Increment(x=w1044) -> (x+1=w1043:i32)
            n403 = Subtract(x=w1049, y="E0 (V vs ref)") -> (x-y=w1021:dbl[])
            n404 = Array Subset(array=w1021, index=w1026, length=w1043) -> (w1018:dbl[])
            n405 = Bundle(w1020, w1021) -> (w1045:cluster{dbl[], dbl[]})  [unwired: 1 in]
            n406 = Array Subset(array=w1020, index=w1026, length=w1043) -> (w1016:dbl[])
            n407 = call <vilib>:"Linear Fit.vi"("Y"=w1018, "X"=w1016) -> ("Best Linear Fit"=w1017:dbl[], "slope"=w1036:dbl, "intercept"=w1042:dbl)  [unwired: 9 in, 2 out]
            n408 = Bundle(w1016, "Best Linear Fit"=w1017) -> (w1019:cluster{dbl[], "Best Linear Fit":dbl[]})  [unwired: 1 in]
            n409 = Build Array(w1045, w1019) -> (w1034:cluster{dbl[], "Best Linear Fit":dbl[]}[])
            n410 = call <vilib>:"Goodness of Fit.vi"("Best Fit"=w1017, "Y"=w1018) -> ("R-square"=→"R² \n[analysis]":dbl)  [unwired: 6 in, 3 out]
            n411 = Divide(x=w1042, y=2.30258509) -> (x/y=w1040:dbl)
            n412 = Power Of 10(x=w1040) -> (10^x=→"i0 (mA)":dbl)
            n413 = Multiply(x=w1036, y=1000.0) -> (x*y=w1038:dbl)
            n414 = Absolute Value(x=w1038) -> (abs(x)=→"Tafel Slope (mV/decade)":dbl)
          }
        }
        "Analysis" <- w971
        n415 = Bundle("error out"=w969, "LINX Resource"=w979) -> (w980:T41)  [unwired: 1 in]
      }
    }
    "Progress" <- w482
    n416 = property on="Current Limit" class="Slide (strict)"() -> ("Scale.Maximum"=w508:dbl, "Scale.Minimum"=w507:dbl)  [unwired: 2 in, 2 out]
    n417 = Unbundle By Name(w495) -> ("error out"=w487:errorcluster)
    n418 = Compound Arithmetic op=OR(w489, w488, w487, "stop") -> (w490:bool)
    n419 = Less Or Equal To 0?(x=w501) -> (x <= 0?=w502:bool)
    n420 = call "Current Limit.vi"("Scale Min"=w507, "Slider Value"=w501, "Scale Max"=w508) -> ("Fill Color"=w506:u32)  [unwired: 8 in]
    n421 = Bundle("Set Current (mA)\n[CP]"=w501, 0.0) -> (→"Current Limit":cluster{"Set Current (mA)\n[CP]":dbl, dbl})  [unwired: 1 in]
    n422 = case shown="True" w502 {
      tunnel: [4 ("Fill Style") 3 ("Fill Style")] -> w503
      frame True {
      }
      frame False {
      }
    }
    n423 = Divide(x=w482, y=60.0 ("x")) -> (x/y=→"time (min)":dbl)
    n424 = property on="Current Limit" class="Slide (strict)"("Fill Color"=w506) -> ()  [unwired: 2 in, 2 out]
    n425 = property on="Current Limit" class="Slide (strict)"("Fill Style"=w503) -> ()  [unwired: 2 in, 2 out]
  }
  n426 = property on="Current Limit" class="Slide (strict)"("Scale.Maximum"=w58, "Scale.Minimum"=w57) -> ()  [unwired: 2 in, 2 out]
  n427 = Unbundle By Name(w37) -> ("Error Out"=w34:errorcluster, "LINX Resource"=w36:T9)
  n428 = call-poly <vilib>:"PWM Set Duty Cycle.vi"("Error In"=w34, "Duty Cycle (0-1)"=w46, "PWM Channel"=u8 9, "LINX Resource"=w36) -> ("Error Out"=w54:errorcluster, "LINX Resource"=w55:T9)  [unwired: 6 in]
  n429 = call-poly <vilib>:"PWM Set Duty Cycle.vi"("Error In"=w54, "Duty Cycle (0-1)"=w46, "PWM Channel"=u8 6, "LINX Resource"=w55) -> ("Error Out"=w48:errorcluster, "LINX Resource"=w51:T9)  [unwired: 6 in]
  n430 = call-poly <vilib>:"PWM Set Duty Cycle.vi"("Error In"=w48, "Duty Cycle (0-1)"=w46, "PWM Channel"=u8 3, "LINX Resource"=w51) -> ("Error Out"=w49:errorcluster, "LINX Resource"=w50:T9)  [unwired: 6 in]
  n431 = call <vilib>:"Close.vi"("Error In"=w49, "LINX Resource"=w50) -> ("Error Out"=w19:errorcluster)  [unwired: 9 in]
  n432 = case shown="False" w45 {
    tunnel: "Method Selector" -> [_ w1055]
    tunnel: w30 -> [_ w1054]
    tunnel: w2 -> [_ w1053]
    tunnel: w19 -> [w1050 w1052]
    tunnel: [w1050 w1051] -> w18
    frame True {
    }
    frame False {
      n433 = case shown="\"Galvanostatic Cycling\"" w1055 {
        tunnel: w1054 -> [w1065 w1088 w1110 w1125 w1135 w1165 w1180 w1199 w1222 w1238 _]
        tunnel: w1053 -> [w1059 w1080 w1104 w1119 w1134 w1164 w1179 w1193 w1217 w1237 _]
        tunnel: w1052 -> [w1058 w1083 w1103 w1118 w1133 w1163 w1178 w1192 w1216 w1236 w1300]
        tunnel: [w1056 w1081 w1101 w1116 w1131 w1161 w1176 w1190 w1214 w1235 w1300] -> w1051
        frame "OCP", Default {
          w1063 = "%#g" ("format (%.3f)")
          n434 = Unbundle By Name(w1059) -> ("Elapsed Time (s)"=w1062:dbl[], "E (V)"=w1061:dbl[])
          n435 = Build Array(w1062, w1061) -> (w1060:dbl[][])
          n436 = call-poly <vilib>:"Write Delimited Spreadsheet.vi"("file path (dialog if empty)"=w1065, "format (%s)"=w1063, "2D data"=string[][] [["Time", "Potential"], ["s", "mV"]], "error in (no error)"=w1058, "delimiter (\\t)"="," ("delimiter (\\t)")) -> ("new file path (Not A Path if cancelled)"=w1067:path, "error out"=w1057:errorcluster)  [unwired: 9 in]
          n437 = call-poly <vilib>:"Write Delimited Spreadsheet.vi"("file path (dialog if empty)"=w1067, "format (%.3f)"=w1063, "2D data"=w1060, "append to file? (new file:F)"=TRUE, "error in (no error)"=w1057, "transpose? (no:F)"=TRUE, "delimiter (\\t)"="," ("delimiter (\\t)")) -> ("error out"=w1056:errorcluster)  [unwired: 7 in, 1 out]
        }
        frame "CV" {
          w1086 = "%#g" ("format (%.3f)")
          n438 = Unbundle By Name(w1080) -> ("E (V)"=w1085:dbl[], "i (mA)"=w1074:dbl[])
          n439 = local read "Cycles\n[CV]"() -> (w1075:i32)
          n440 = Array Size(array=w1074) -> (size(s)=w1079:i32)
          n441 = To Double Precision Float(number=w1075) -> (double precision float=w1077:dbl)
          n442 = To Double Precision Float(number=w1079) -> (double precision float=w1078:dbl)
          n443 = Divide(x=w1078, y=w1077) -> (x/y=w1076:dbl)
          n444 = for {
            N: w1075 -> [_]
            tunnel: w1076 -> [w1098]
            shift-right: [w1096] -> w1072
            shift-left: i32[] [] -> [w1095]
            i -> [w1100]
            n445 = Increment(x=w1100) -> (x+1=w1099:i32)
            n446 = To Long Integer(number=w1098) -> (32bit integer=w1097:i32)
            n447 = Initialize Array(w1099, w1097) -> (w1094:i32[])
            n448 = Insert Into Array(array=w1095, new element=w1094) -> (w1096:i32[])  [unwired: 1 in]
          }
          n449 = To Double Precision Float(number=w1072) -> (double precision float=w1071:dbl[])
          n450 = Build Array(w1085, w1074, w1071) -> (w1084:dbl[][])
          n451 = call-poly <vilib>:"Write Delimited Spreadsheet.vi"("file path (dialog if empty)"=w1088, "format (%s)"=w1086, "2D data"=string[][] [["Potential", "Current", "Cycle", ""], ["V vs ref", "mA", "#", ""]], "error in (no error)"=w1083, "delimiter (\\t)"="," ("delimiter (\\t)")) -> ("new file path (Not A Path if cancelled)"=w1090:path, "error out"=w1082:errorcluster)  [unwired: 9 in]
          n452 = call-poly <vilib>:"Write Delimited Spreadsheet.vi"("file path (dialog if empty)"=w1090, "format (%.3f)"=w1086, "2D data"=w1084, "append to file? (new file:F)"=TRUE, "error in (no error)"=w1082, "transpose? (no:F)"=TRUE, "delimiter (\\t)"="," ("delimiter (\\t)")) -> ("error out"=w1081:errorcluster)  [unwired: 7 in, 1 out]
        }
        frame "LSV" {
          w1108 = "%#g" ("format (%.3f)")
          n453 = Unbundle By Name(w1104) -> ("E (V)"=w1107:dbl[], "i (mA)"=w1106:dbl[])
          n454 = Build Array(w1107, w1106) -> (w1105:dbl[][])
          n455 = call-poly <vilib>:"Write Delimited Spreadsheet.vi"("file path (dialog if empty)"=w1110, "format (%s)"=w1108, "2D data"=string[][] [["Potential", "Current", "", ""], ["V vs ref", "mA", "", ""]], "error in (no error)"=w1103, "delimiter (\\t)"="," ("delimiter (\\t)")) -> ("new file path (Not A Path if cancelled)"=w1112:path, "error out"=w1102:errorcluster)  [unwired: 9 in]
          n456 = call-poly <vilib>:"Write Delimited Spreadsheet.vi"("file path (dialog if empty)"=w1112, "format (%.3f)"=w1108, "2D data"=w1105, "append to file? (new file:F)"=TRUE, "error in (no error)"=w1102, "transpose? (no:F)"=TRUE, "delimiter (\\t)"="," ("delimiter (\\t)")) -> ("error out"=w1101:errorcluster)  [unwired: 7 in, 1 out]
        }
        frame "ASV" {
          w1123 = "%#g" ("format (%.3f)")
          n457 = Unbundle By Name(w1119) -> ("E (V)"=w1122:dbl[], "i (mA)"=w1121:dbl[])
          n458 = Build Array(w1122, w1121) -> (w1120:dbl[][])
          n459 = call-poly <vilib>:"Write Delimited Spreadsheet.vi"("file path (dialog if empty)"=w1125, "format (%s)"=w1123, "2D data"=string[][] [["Potential", "Current", "", ""], ["V vs ref", "mA", "", ""]], "error in (no error)"=w1118, "delimiter (\\t)"="," ("delimiter (\\t)")) -> ("new file path (Not A Path if cancelled)"=w1127:path, "error out"=w1117:errorcluster)  [unwired: 9 in]
          n460 = call-poly <vilib>:"Write Delimited Spreadsheet.vi"("file path (dialog if empty)"=w1127, "format (%.3f)"=w1123, "2D data"=w1120, "append to file? (new file:F)"=TRUE, "error in (no error)"=w1117, "transpose? (no:F)"=TRUE, "delimiter (\\t)"="," ("delimiter (\\t)")) -> ("error out"=w1116:errorcluster)  [unwired: 7 in, 1 out]
        }
        frame "CA" {
          w1149 = "%#g" ("format (%.3f)")
          # "s wait time"
          n461 = Unbundle By Name(w1134) -> ("Elapsed Time (s)"=w1143:dbl[], "i (mA)"=w1144:dbl[])
          n462 = Index Array(array=w1143, index #1=2 ("index"), index #2=1 ("index")) -> (element #1=w1139:dbl, element #2=w1140:dbl)
          n463 = Subtract(x=w1139, y=w1140) -> (x-y=w1137:dbl)
          n464 = Multiply(x=w1137, y=1000.0) -> (x*y=w1136:dbl)
          n465 = call <vilib>:"Integral x(t).vi"("dt"=w1136, "X"=w1144) -> ("Integral X"=w1146:dbl[])  [unwired: 8 in, 1 out]
          n466 = call-poly <vilib>:"Write Delimited Spreadsheet.vi"("file path (dialog if empty)"=w1135, "format (%s)"=w1149, "2D data"=string[][] [["Time", "Current", "Charge"], ["s", "mA", "C"]], "error in (no error)"=w1133, "delimiter (\\t)"="," ("delimiter (\\t)")) -> ("new file path (Not A Path if cancelled)"=w1152:path, "error out"=w1132:errorcluster)  [unwired: 9 in]
          n467 = Divide(x=w1146, y=1000000.0) -> (x/y=w1145:dbl[])
          n468 = Build Array(w1143, w1144, w1145) -> (w1148:dbl[][])
          n469 = call-poly <vilib>:"Write Delimited Spreadsheet.vi"("file path (dialog if empty)"=w1152, "format (%.3f)"=w1149, "2D data"=w1148, "append to file? (new file:F)"=TRUE, "error in (no error)"=w1132, "transpose? (no:F)"=TRUE, "delimiter (\\t)"="," ("delimiter (\\t)")) -> ("error out"=w1131:errorcluster)  [unwired: 7 in, 1 out]
        }
        frame "CP" {
          w1168 = "%#g" ("format (%.3f)")
          n470 = local read "Set Current (mA)\n[CP]"() -> (w1159:dbl)
          n471 = Unbundle By Name(w1164) -> ("Elapsed Time (s)"=w1160:dbl[], "Eraw (V)"=w1166:dbl[])
          n472 = Multiply(x=w1160, y=w1159) -> (x*y=w1157:dbl[])
          n473 = Divide(x=w1157, y=1000.0) -> (x/y=w1156:dbl[])
          n474 = call-poly <vilib>:"Write Delimited Spreadsheet.vi"("file path (dialog if empty)"=w1165, "format (%s)"=w1168, "2D data"=string[][] [["Time", "Potential", "Charge"], ["s", "V", "C"]], "error in (no error)"=w1163, "delimiter (\\t)"="," ("delimiter (\\t)")) -> ("new file path (Not A Path if cancelled)"=w1171:path, "error out"=w1162:errorcluster)  [unwired: 9 in]
          n475 = Build Array(w1160, w1166, w1156) -> (w1167:dbl[][])
          n476 = call-poly <vilib>:"Write Delimited Spreadsheet.vi"("file path (dialog if empty)"=w1171, "format (%.3f)"=w1168, "2D data"=w1167, "append to file? (new file:F)"=TRUE, "error in (no error)"=w1162, "transpose? (no:F)"=TRUE, "delimiter (\\t)"="," ("delimiter (\\t)")) -> ("error out"=w1161:errorcluster)  [unwired: 7 in, 1 out]
        }
        frame "Galvanostatic Cycling" {
          w1183 = "%#g" ("format (%.3f)")
          n477 = Unbundle By Name(w1179) -> ("Elapsed Time (s)"=w1175:dbl[], "Eraw (V)"=w1181:dbl[])
          n478 = call-poly <vilib>:"Write Delimited Spreadsheet.vi"("file path (dialog if empty)"=w1180, "format (%s)"=w1183, "2D data"=string[][] [["Time", "Potential", ""], ["s", "V", ""]], "error in (no error)"=w1178, "delimiter (\\t)"="," ("delimiter (\\t)")) -> ("new file path (Not A Path if cancelled)"=w1186:path, "error out"=w1177:errorcluster)  [unwired: 9 in]
          n479 = Build Array(w1175, w1181) -> (w1182:dbl[][])
          n480 = call-poly <vilib>:"Write Delimited Spreadsheet.vi"("file path (dialog if empty)"=w1186, "format (%.3f)"=w1183, "2D data"=w1182, "append to file? (new file:F)"=TRUE, "error in (no error)"=w1177, "transpose? (no:F)"=TRUE, "delimiter (\\t)"="," ("delimiter (\\t)")) -> ("error out"=w1176:errorcluster)  [unwired: 7 in, 1 out]
        }
        frame "Ohmic Drop" {
          w1197 = "%#g" ("format (%.3f)")
          n481 = Unbundle By Name(w1193) -> ("Elapsed Time (s)"=w1196:dbl[], "i (mA)"=w1195:dbl[])
          n482 = Build Array(w1196, w1195) -> (w1194:dbl[][])
          n483 = call-poly <vilib>:"Write Delimited Spreadsheet.vi"("file path (dialog if empty)"=w1199, "format (%s)"=w1197, "2D data"=string[][] [["Time", "Current", "", ""], ["s", "mA", "", ""]], "error in (no error)"=w1192, "delimiter (\\t)"="," ("delimiter (\\t)")) -> ("new file path (Not A Path if cancelled)"=w1201:path, "error out"=w1191:errorcluster)  [unwired: 9 in]
          n484 = call-poly <vilib>:"Write Delimited Spreadsheet.vi"("file path (dialog if empty)"=w1201, "format (%.3f)"=w1197, "2D data"=w1194, "append to file? (new file:F)"=TRUE, "error in (no error)"=w1191, "transpose? (no:F)"=TRUE, "delimiter (\\t)"="," ("delimiter (\\t)")) -> ("error out"=w1190:errorcluster)  [unwired: 7 in, 1 out]
        }
        frame "Calibration" {
          w1220 = "%#g" ("format (%.3f)")
          n485 = local read "Cycles \n[Cal]"() -> (w1205:i32)
          n486 = Unbundle By Name(w1217) -> ("Eraw (V)"=w1219:dbl[], "Vr (V)"=w1206:dbl[])
          n487 = Array Size(array=w1206) -> (size(s)=w1213:i32)
          n488 = To Double Precision Float(number=w1205) -> (double precision float=w1211:dbl)
          n489 = To Double Precision Float(number=w1213) -> (double precision float=w1212:dbl)
          n490 = Divide(x=w1212, y=w1211) -> (x/y=w1210:dbl)
          n491 = for {
            N: w1205 -> [_]
            tunnel: w1210 -> [w1232]
            shift-right: [w1230] -> w1208
            shift-left: i32[] [] -> [w1229]
            i -> [w1234]
            n492 = To Long Integer(number=w1232) -> (32bit integer=w1231:i32)
            n493 = Increment(x=w1234) -> (x+1=w1233:i32)
            n494 = Initialize Array(w1233, w1231) -> (w1228:i32[])
            n495 = Insert Into Array(array=w1229, new element=w1228) -> (w1230:i32[])  [unwired: 1 in]
          }
          n496 = To Double Precision Float(number=w1208) -> (double precision float=w1207:dbl[])
          n497 = Build Array(w1219, w1206, w1207) -> (w1218:dbl[][])
          n498 = call-poly <vilib>:"Write Delimited Spreadsheet.vi"("file path (dialog if empty)"=w1222, "format (%s)"=w1220, "2D data"=string[][] [["Potential", "Response Voltage", "Cycle"], ["V vs ref", "V", "#"]], "error in (no error)"=w1216, "delimiter (\\t)"="," ("delimiter (\\t)")) -> ("new file path (Not A Path if cancelled)"=w1224:path, "error out"=w1215:errorcluster)  [unwired: 9 in]
          n499 = call-poly <vilib>:"Write Delimited Spreadsheet.vi"("file path (dialog if empty)"=w1224, "format (%.3f)"=w1220, "2D data"=w1218, "append to file? (new file:F)"=TRUE, "error in (no error)"=w1215, "transpose? (no:F)"=TRUE, "delimiter (\\t)"="," ("delimiter (\\t)")) -> ("error out"=w1214:errorcluster)  [unwired: 7 in, 1 out]
        }
        frame "Method Builder" {
          n500 = case shown="1" "Save Plot" {
            tunnel: w1238 -> [w1255 w1285]
            tunnel: w1237 -> [w1252 w1282]
            tunnel: w1236 -> [w1251 w1279]
            tunnel: [w1249 w1281] -> w1235
            frame 0, Default {
              w1256 = "%#g" ("format (%.3f)")
              n501 = local read "Cycles\n[MB]"() -> (w1240:i32)
              n502 = Unbundle By Name(w1252) -> ("E (V)"=w1254:dbl[], "i (mA)"=w1241:dbl[])
              n503 = Array Size(array=w1241) -> (size(s)=w1248:i32)
              n504 = To Double Precision Float(number=w1248) -> (double precision float=w1247:dbl)
              n505 = To Double Precision Float(number=w1240) -> (double precision float=w1246:dbl)
              n506 = Divide(x=w1247, y=w1246) -> (x/y=w1245:dbl)
              n507 = for {
                N: w1240 -> [_]
                tunnel: w1245 -> [w1267]
                shift-right: [w1265] -> w1243
                shift-left: i32[] [] -> [w1264]
                i -> [w1269]
                n508 = Increment(x=w1269) -> (x+1=w1268:i32)
                n509 = To Long Integer(number=w1267) -> (32bit integer=w1266:i32)
                n510 = Initialize Array(w1268, w1266) -> (w1263:i32[])
                n511 = Insert Into Array(array=w1264, new element=w1263) -> (w1265:i32[])  [unwired: 1 in]
              }
              n512 = To Double Precision Float(number=w1243) -> (double precision float=w1242:dbl[])
              n513 = Build Array(w1254, w1241, w1242) -> (w1253:dbl[][])
              n514 = call-poly <vilib>:"Write Delimited Spreadsheet.vi"("file path (dialog if empty)"=w1255, "format (%s)"=w1256, "2D data"=string[][] [["Potential", "Current", "Cycle"], ["V vs ref", "mA", "1"]], "error in (no error)"=w1251, "delimiter (\\t)"="," ("delimiter (\\t)")) -> ("new file path (Not A Path if cancelled)"=w1259:path, "error out"=w1250:errorcluster)  [unwired: 9 in]
              n515 = call-poly <vilib>:"Write Delimited Spreadsheet.vi"("file path (dialog if empty)"=w1259, "format (%.3f)"=w1256, "2D data"=w1253, "append to file? (new file:F)"=TRUE, "error in (no error)"=w1250, "transpose? (no:F)"=TRUE, "delimiter (\\t)"="," ("delimiter (\\t)")) -> ("error out"=w1249:errorcluster)  [unwired: 7 in, 1 out]
            }
            frame 1 {
              w1286 = "%#g" ("format (%.3f)")
              n516 = local read "Cycles\n[MB]"() -> (w1271:i32)
              n517 = Unbundle By Name(w1282) -> ("Elapsed Time (s)"=w1284:dbl[], "i (mA)"=w1272:dbl[])
              n518 = Array Size(array=w1272) -> (size(s)=w1278:i32)
              n519 = To Double Precision Float(number=w1278) -> (double precision float=w1277:dbl)
              n520 = To Double Precision Float(number=w1271) -> (double precision float=w1276:dbl)
              n521 = Divide(x=w1277, y=w1276) -> (x/y=w1275:dbl)
              n522 = for {
                N: w1271 -> [_]
                tunnel: w1275 -> [w1297]
                shift-right: [w1295] -> w1273
                shift-left: i32[] [] -> [w1294]
                i -> [w1299]
                n523 = Increment(x=w1299) -> (x+1=w1298:i32)
                n524 = To Long Integer(number=w1297) -> (32bit integer=w1296:i32)
                n525 = Initialize Array(w1298, w1296) -> (w1293:i32[])
                n526 = Insert Into Array(array=w1294, new element=w1293) -> (w1295:i32[])  [unwired: 1 in]
              }
              n527 = To Double Precision Float(number=w1273) -> (double precision float=w1270:dbl[])
              n528 = Build Array(w1284, w1272, w1270) -> (w1283:dbl[][])
              n529 = call-poly <vilib>:"Write Delimited Spreadsheet.vi"("file path (dialog if empty)"=w1285, "format (%s)"=w1286, "2D data"=string[][] [["Time", "Current", "Cycle"], ["s", "mA", "#"]], "error in (no error)"=w1279, "delimiter (\\t)"="," ("delimiter (\\t)")) -> ("new file path (Not A Path if cancelled)"=w1289:path, "error out"=w1280:errorcluster)  [unwired: 9 in]
              n530 = call-poly <vilib>:"Write Delimited Spreadsheet.vi"("file path (dialog if empty)"=w1289, "format (%.3f)"=w1286, "2D data"=w1283, "append to file? (new file:F)"=TRUE, "error in (no error)"=w1280, "transpose? (no:F)"=TRUE, "delimiter (\\t)"="," ("delimiter (\\t)")) -> ("error out"=w1281:errorcluster)  [unwired: 7 in, 1 out]
            }
          }
        }
        frame "Analysis" {
        }
      }
    }
  }
  n531 = case shown="\"Galvanostatic Cycling\"" "Method Selector" {
    tunnel: [w1301 w1302 w1303 w1304 w1305 w1306 w1307 w1308 w1312 w1313 w1314] -> w31
    tunnel: w18 -> [w1301 w1302 w1303 w1304 w1305 w1306 w1307 w1308 w1311 w1313 w1314]
    tunnel: w12 -> [_ _ _ _ _ _ _ _ w1309 _ _]
    frame "OCP", Default {
    }
    frame "CV" {
    }
    frame "LSV" {
    }
    frame "ASV" {
    }
    frame "CA" {
    }
    frame "CP" {
    }
    frame "Galvanostatic Cycling" {
    }
    frame "Ohmic Drop" {
    }
    frame "Calibration" {
      n532 = call <vilib>:"Application Directory.vi"() -> ("Application Directory"=w1310:path)
      n533 = call "Write INI.vi"("Conversion and Correction"=w1309, "error in (no error)"=w1311, "Path"=w1310) -> ("error out"=w1312:errorcluster)
    }
    frame "Method Builder" {
    }
    frame "Analysis" {
    }
  }
  n534 = call <vilib>:"Simple Error Handler.vi"("error in (no error)"=w31) -> ()  [unwired: 4 in, 5 out]
